vi "TXRX 5785 DDC DUC Measure Phase Stability.vi"() -> (0 "error out":errorcluster)   [LabVIEW 2019]
uses:
  <vilib>/userDefined/Silver/nirio_resource_slv.ctl
  <instrlib>/FlexRIO/API/Host/v1/NI FlexRIO/API/Reference Clock Source.ctl
  Common/Original 5785 Example/Host/Upconversion Mode.ctl
  <vilib>/Analysis/1siggen.llb/Ramp Pattern by Delta.vi
  <instrlib>/FlexRIO/API/Host/v1/NI FlexRIO/API/Configure Reference Clock.vi
  <instrlib>/FlexRIO/API/Host/v1/NI FlexRIO/API/Get Property Reference - Fpga Small.vi
  <instrlib>/FlexRIO/API/Host/v1/NI FlexRIO/API/Configure Analog Start Trigger.vi
  <instrlib>/FlexRIO/API/Host/v1/NI FlexRIO/API/Configure Digital Edge Start Trigger.vi
  <instrlib>/FlexRIO/API/Host/v1/NI FlexRIO/API/Configure Immediate Start Trigger.vi
  <instrlib>/FlexRIO/API/Host/v1/NI FlexRIO/API/Read Stream 1D WDT.vi
  <vilib>/measure/maspectr.llb/FFT Power Spectrum and PSD for N Chan.vi
  <vilib>/FPGAPlugInAG/Dynamic/niLvFpga_Close_Dynamic.vi
  <vilib>/Utility/file.llb/Write Delimited Spreadsheet (string).vi
  <vilib>/rvi/interface/nirviCloseFPGA/nirviCloseFPGA.xnode
  <instrlib>/FlexRIO/API/Host/v1/NI FlexRIO API v1.lvlib
  <resource>/objmgr/niflexrioapiStream.rc
  <vilib>/measure/NI_MAPro.lvlib
  Common/Original 5785 Example/Host/GettingStarted_5785_Host.lvlib
  <vilib>/Analysis/NI_AALPro.lvlib
  <vilib>/Analysis/NI_AALBase.lvlib
  <vilib>/measure/matone.llb/Extract Single Tone Information N Chan.vi
panel:
  out "Magnitude":cluster{"t0":dbl, "dt":dbl, "Y":dbl[]}(graph)={"t0"=0.0, "dt"=6.25e-10, "Y"=[0.00021584455710773213, 0.00043168911421546426, 0.00043168911421546426, 0.0004826431022662244, 0.00021584455710773213, 0.00021584455710773213, 0.0, 0.0003052503000261688, 0.00021584455710773213, 0.0003052503000261688, 0.0003052503000261688, 0.00021584455710773213, 0.0008899499076698426, 0.0004826431022662244, 0.00021584455710773213, 0.0004826431022662244, 0.00021584455710773213, 0.0004826431022662244, 0.00021584455710773213, 0.0006825604210107193, 0.00021584455710773213, 0.00021584455710773213, 0.0003052503000261688, 0.00021584455710773213, 0.00043168911421546426, 0.0004826431022662244, 0.0004826431022662244, 0.00043168911421546426, 0.0006825604210107193, 0.0004826431022662244, 0.00021584455710773213, 0.0006475336713231963, 0.00043168911421546426, 0.00021584455710773213, 0.0, 0.0003052503000261688, 0.0003052503000261688, 0.00021584455710773213, 0.0003052503000261688, 0.0003052503000261688, 0.0, 0.0, 0.00043168911421546426, 0.0004826431022662244, 0.00043168911421546426, 0.00043168911421546426, 0.0007782386181817434, 0.00021584455710773213, 0.00021584455710773213, 0.0003052503000261688, 0.00021584455710773213, 0.0, 0.00021584455710773213, 0.0003052503000261688, 0.00021584455710773213, 0.0004826431022662244, 0.00043168911421546426, 0.00043168911421546426, 0.0004826431022662244, 0.0003052503000261688, 0.0003052503000261688, 0.0004826431022662244, 0.0006825604210107193, 0.0004826431022662244, 0.00043168911421546426, 0.0003052503000261688, 0.0003052503000261688, 0.0003052503000261688, 0.00043168911421546426, 0.0004826431022662244, 0.0006825604210107193, 0.0003052503000261688, 0.0003052503000261688, 0.0, 0.00021584455710773213, 0.0003052503000261688, 0.0003052503000261688, 0.0004826431022662244, 0.0003052503000261688, 0.00021584455710773213, 0.00021584455710773213, 0.0011623585127480927, 0.0003052503000261688, 0.0006825604210107193, 0.00021584455710773213, 0.00021584455710773213, 0.00021584455710773213, 0.0006475336713231963, 0.0004826431022662244, 0.0004826431022662244, 0.0, 0.0003052503000261688, 0.00021584455710773213, 0.00021584455710773213, 0.00021584455710773213, 0.00021584455710773213, 0.0, 0.00021584455710773213, 0.00021584455710773213, 0.00043168911421546426, 0.0004826431022662244, 0.00021584455710773213, 0.0003052503000261688, 0.0, 0.00021584455710773213, 0.0003052503000261688, 0.0, 0.0003052503000261688, 0.0004826431022662244, 0.00021584455710773213, 0.0006105006000523376, 0.0003052503000261688, 0.00043168911421546426, 0.0, 0.00021584455710773213, 0.00043168911421546426, 0.0003052503000261688, 0.0, 0.00043168911421546426, 0.00021584455710773213, 0.0003052503000261688, 0.00021584455710773213, 0.00021584455710773213, 0.0004826431022662244, 0.0006105006000523376, 0.0003052503000261688, 0.0006105006000523376, 0.00021584455710773213, 0.0, 0.0004826431022662244, 0.00021584455710773213, 0.00021584455710773213, 0.0003052503000261688, 0.00021584455710773213, 0.00021584455710773213, 0.0004826431022662244, 0.00021584455710773213, 0.0004826431022662244, 0.00021584455710773213, 0.0004826431022662244, 0.0003052503000261688, 0.0, 0.0007782386181817434, 0.00021584455710773213, 0.00021584455710773213, 0.00043168911421546426, 0.00021584455710773213, 0.0, 0.00021584455710773213, 0.00021584455710773213, 0.00021584455710773213, 0.0003052503000261688, 0.00021584455710773213, 0.00043168911421546426, 0.0004826431022662244, 0.00021584455710773213, 0.0004826431022662244, 0.0003052503000261688, 0.0004826431022662244, 0.0003052503000261688, 0.0, 0.00021584455710773213, 0.00021584455710773213, 0.00043168911421546426, 0.0003052503000261688, 0.00021584455710773213, 0.0004826431022662244, 0.0003052503000261688, 0.00021584455710773213, 0.0, 0.0003052503000261688, 0.0004826431022662244, 0.0006825604210107193, 0.0, 0.00021584455710773213, 0.0, 0.0, 0.0, 0.0003052503000261688, 0.00021584455710773213, 0.00043168911421546426, 0.0004826431022662244, 0.0, 0.00021584455710773213, 0.0006105006000523376, 0.0004826431022662244, 0.00021584455710773213, 0.00021584455710773213, 0.0003052503000261688, 0.0003052503000261688, 0.0004826431022662244, 0.0, 0.00043168911421546426, 0.0004826431022662244, 0.00021584455710773213, 0.0003052503000261688, 0.0, 0.0, 0.00021584455710773213, 0.00021584455710773213, 0.00021584455710773213, 0.00021584455710773213, 0.0003052503000261688, 0.00021584455710773213, 0.00021584455710773213, 0.00021584455710773213, 0.0003052503000261688, 0.0003052503000261688, 0.00021584455710773213, 0.00021584455710773213, 0.00043168911421546426, 0.00021584455710773213, 0.0003052503000261688, 0.00021584455710773213, 0.0006475336713231963, 0.0, 0.0003052503000261688, 0.00021584455710773213, 0.0, 0.00021584455710773213, 0.00021584455710773213, 0.00021584455710773213, 0.00021584455710773213, 0.00043168911421546426, 0.0003052503000261688, 0.0006475336713231963, 0.0, 0.00043168911421546426, 0.0006475336713231963, 0.0003052503000261688, 0.0006825604210107193, 0.0003052503000261688, 0.0003052503000261688, 0.00021584455710773213, 0.0, 0.0003052503000261688, 0.0004826431022662244, 0.00021584455710773213, 0.0004826431022662244, 0.0006825604210107193, 0.00021584455710773213, 0.00043168911421546426, 0.00021584455710773213, 0.00021584455710773213, 0.0006475336713231963, 0.00021584455710773213, 0.0004826431022662244, 0.00021584455710773213, 0.0, 0.0008899499076698426, 0.00021584455710773213, 0.00043168911421546426, 0.0006105006000523376, 0.00021584455710773213, 0.0006105006000523376, 0.0003052503000261688, 0.00021584455710773213, 0.0006475336713231963, 0.0003052503000261688, 0.0003052503000261688, 0.0003052503000261688, 0.00021584455710773213, 0.0003052503000261688, 0.0003052503000261688, 0.0004826431022662244, 0.00021584455710773213, 0.00021584455710773213, 0.00043168911421546426, 0.00043168911421546426, 0.00021584455710773213, 0.0, 0.00021584455710773213, 0.00021584455710773213, 0.00043168911421546426, 0.0003052503000261688, 0.00021584455710773213, 0.00021584455710773213, 0.00043168911421546426, 0.0003052503000261688, 0.00043168911421546426, 0.00021584455710773213, 0.00021584455710773213, 0.0004826431022662244, 0.0004826431022662244, 0.00043168911421546426, 0.00021584455710773213, 0.00021584455710773213, 0.0003052503000261688, 0.0, 0.0, 0.00043168911421546426, 0.0003052503000261688, 0.00021584455710773213, 0.0004826431022662244, 0.00021584455710773213, 0.0, 0.00021584455710773213, 0.00021584455710773213, 0.00021584455710773213, 0.00043168911421546426, 0.0004826431022662244, 0.0003052503000261688, 0.00043168911421546426, 0.0003052503000261688, 0.00021584455710773213, 0.0, 0.00021584455710773213, 0.0003052503000261688, 0.0, 0.00021584455710773213, 0.0004826431022662244, 0.0009157509000785064, 0.00021584455710773213, 0.0007782386181817434, 0.00021584455710773213, 0.0, 0.00021584455710773213, 0.0003052503000261688, 0.00043168911421546426, 0.0004826431022662244, 0.0003052503000261688, 0.00021584455710773213, 0.0003052503000261688, 0.00021584455710773213, 0.00021584455710773213, 0.0, 0.0003052503000261688, 0.0003052503000261688, 0.00021584455710773213, 0.0003052503000261688, 0.00021584455710773213, 0.00043168911421546426, 0.00043168911421546426, 0.0003052503000261688, 0.0003052503000261688, 0.00021584455710773213, 0.00021584455710773213, 0.0003052503000261688, 0.00021584455710773213, 0.00021584455710773213, 0.0003052503000261688, 0.0003052503000261688, 0.0004826431022662244, 0.00021584455710773213, 0.0004826431022662244, 0.0004826431022662244, 0.00021584455710773213, 0.00043168911421546426, 0.0004826431022662244, 0.0004826431022662244, 0.0003052503000261688, 0.00043168911421546426, 0.00043168911421546426, 0.0006825604210107193, 0.00021584455710773213, 0.00021584455710773213, 0.0, 0.0004826431022662244, 0.00043168911421546426, 0.00021584455710773213, 0.0, 0.0003052503000261688, 0.00021584455710773213, 0.00043168911421546426, 0.0003052503000261688, 0.00021584455710773213, 0.0006825604210107193, 0.00021584455710773213, 0.00021584455710773213, 0.00021584455710773213, 0.00021584455710773213, 0.0003052503000261688, 0.0004826431022662244, 0.00021584455710773213, 0.0, 0.00021584455710773213, 0.0003052503000261688, 0.0004826431022662244, 0.0006475336713231963, 0.0003052503000261688, 0.00043168911421546426, 0.0, 0.0004826431022662244, 0.00021584455710773213, 0.0003052503000261688, 0.00021584455710773213, 0.0004826431022662244, 0.0003052503000261688, 0.00021584455710773213, 0.00021584455710773213, 0.0003052503000261688, 0.0003052503000261688, 0.0003052503000261688, 0.00043168911421546426, 0.0003052503000261688, 0.0, 0.00021584455710773213, 0.0003052503000261688, 0.00021584455710773213, 0.00021584455710773213, 0.0004826431022662244, 0.00043168911421546426, 0.00021584455710773213, 0.0003052503000261688, 0.0, 0.0003052503000261688, 0.0004826431022662244, 0.0003052503000261688, 0.00021584455710773213, 0.00021584455710773213, 0.00021584455710773213, 0.00021584455710773213, 0.00021584455710773213, 0.00021584455710773213, 0.0003052503000261688, 0.00021584455710773213, 0.0003052503000261688, 0.0003052503000261688, 0.0, 0.0, 0.0, 0.0003052503000261688, 0.00021584455710773213, 0.0004826431022662244, 0.0006475336713231963, 0.0006825604210107193, 0.00021584455710773213, 0.00021584455710773213, 0.00043168911421546426, 0.00021584455710773213, 0.00021584455710773213, 0.0003052503000261688, 0.0004826431022662244, 0.0004826431022662244, 0.00021584455710773213, 0.0, 0.0, 0.0003052503000261688, 0.0004826431022662244, 0.00021584455710773213, 0.0003052503000261688, 0.0004826431022662244, 0.00021584455710773213, 0.0003052503000261688, 0.00021584455710773213, 0.0003052503000261688, 0.0004826431022662244, 0.00021584455710773213, 0.0004826431022662244, 0.00021584455710773213, 0.0003052503000261688, 0.0003052503000261688, 0.0004826431022662244, 0.0, 0.00021584455710773213, 0.0, 0.00043168911421546426, 0.00043168911421546426, 0.0004826431022662244, 0.00043168911421546426, 0.00043168911421546426, 0.00021584455710773213, 0.00021584455710773213, 0.0004826431022662244, 0.00021584455710773213, 0.00021584455710773213, 0.00021584455710773213, 0.00021584455710773213, 0.00021584455710773213, 0.0004826431022662244, 0.0003052503000261688, 0.0004826431022662244, 0.0004826431022662244, 0.0006105006000523376, 0.0003052503000261688, 0.0, 0.0003052503000261688, 0.0003052503000261688, 0.0004826431022662244, 0.0004826431022662244, 0.00043168911421546426, 0.0004826431022662244, 0.0, 0.0, 0.0003052503000261688, 0.0003052503000261688, 0.0, 0.00021584455710773213, 0.00021584455710773213, 0.0003052503000261688, 0.00021584455710773213, 0.0003052503000261688, 0.00021584455710773213, 0.0003052503000261688, 0.00021584455710773213, 0.0003052503000261688, 0.00043168911421546426, 0.0004826431022662244, 0.00021584455710773213, 0.0003052503000261688, 0.00021584455710773213, 0.0003052503000261688, 0.0003052503000261688, 0.00021584455710773213, 0.00043168911421546426, 0.0003052503000261688, 0.0, 0.00021584455710773213, 0.0004826431022662244, 0.0003052503000261688, 0.0006105006000523376, 0.00021584455710773213, 0.0004826431022662244, 0.00021584455710773213, 0.00021584455710773213, 0.00021584455710773213, 0.0, 0.00021584455710773213, 0.0004826431022662244, 0.00021584455710773213, 0.0003052503000261688, 0.00021584455710773213, 0.0006825604210107193, 0.0003052503000261688, 0.0003052503000261688, 0.0003052503000261688, 0.0003052503000261688, 0.00021584455710773213, 0.0003052503000261688, 0.0, 0.00043168911421546426, 0.0003052503000261688, 0.0003052503000261688, 0.0003052503000261688, 0.00021584455710773213, 0.0003052503000261688, 0.0003052503000261688, 0.00043168911421546426, 0.0003052503000261688, 0.0003052503000261688, 0.0004826431022662244, 0.00021584455710773213, 0.0, 0.0003052503000261688, 0.0003052503000261688, 0.0004826431022662244, 0.00043168911421546426, 0.0003052503000261688, 0.00021584455710773213, 0.0, 0.0006105006000523376, 0.0004826431022662244, 0.00021584455710773213, 0.00021584455710773213, 0.0003052503000261688, 0.0004826431022662244, 0.0003052503000261688, 0.00043168911421546426, 0.0003052503000261688, 0.0004826431022662244, 0.0003052503000261688, 0.0006825604210107193, 0.0, 0.00021584455710773213, 0.0003052503000261688, 0.00021584455710773213, 0.0, 0.0, 0.00021584455710773213, 0.00021584455710773213, 0.0, 0.0004826431022662244, 0.0003052503000261688, 0.00021584455710773213, 0.0, 0.0, 0.00021584455710773213, 0.0003052503000261688, 0.0003052503000261688, 0.00021584455710773213, 0.00021584455710773213, 0.0004826431022662244, 0.00021584455710773213, 0.0003052503000261688, 0.00021584455710773213, 0.0004826431022662244, 0.00021584455710773213, 0.0004826431022662244, 0.0003052503000261688, 0.00021584455710773213, 0.0, 0.0003052503000261688, 0.0003052503000261688, 0.0003052503000261688, 0.0, 0.00043168911421546426, 0.0004826431022662244, 0.0, 0.0003052503000261688, 0.00021584455710773213, 0.0006105006000523376, 0.0004826431022662244, 0.00021584455710773213, 0.0003052503000261688, 0.0003052503000261688, 0.0003052503000261688, 0.0, 0.0003052503000261688, 0.0004826431022662244, 0.00021584455710773213, 0.00021584455710773213, 0.0004826431022662244, 0.00043168911421546426, 0.0, 0.0004826431022662244, 0.00021584455710773213, 0.0003052503000261688, 0.0, 0.00021584455710773213, 0.00021584455710773213, 0.0003052503000261688, 0.0003052503000261688, 0.00021584455710773213, 0.00043168911421546426, 0.00021584455710773213, 0.00021584455710773213, 0.0004826431022662244, 0.0003052503000261688, 0.0004826431022662244, 0.0004826431022662244, 0.00021584455710773213, 0.0004826431022662244, 0.00021584455710773213, 0.0, 0.0006475336713231963, 0.0, 0.00021584455710773213, 0.0, 0.0004826431022662244, 0.00043168911421546426, 0.0, 0.0, 0.0006105006000523376, 0.00021584455710773213, 0.00021584455710773213, 0.0003052503000261688, 0.0004826431022662244, 0.00021584455710773213, 0.0003052503000261688, 0.0, 0.0003052503000261688, 0.0004826431022662244, 0.0004826431022662244, 0.0004826431022662244, 0.0004826431022662244, 0.0004826431022662244, 0.00021584455710773213, 0.0, 0.00021584455710773213, 0.00021584455710773213, 0.00021584455710773213, 0.0004826431022662244, 0.00021584455710773213, 0.0003052503000261688, 0.0003052503000261688, 0.00043168911421546426, 0.00021584455710773213, 0.0003052503000261688, 0.0004826431022662244, 0.0003052503000261688, 0.0003052503000261688, 0.00043168911421546426, 0.00021584455710773213, 0.0003052503000261688, 0.0004826431022662244, 0.0003052503000261688, 0.0006825604210107193, 0.00043168911421546426, 0.00021584455710773213, 0.0003052503000261688, 0.0003052503000261688, 0.00021584455710773213, 0.0, 0.00021584455710773213, 0.0003052503000261688, 0.0, 0.0004826431022662244, 0.00021584455710773213, 0.00021584455710773213, 0.0004826431022662244, 0.00021584455710773213, 0.0003052503000261688, 0.00021584455710773213, 0.0003052503000261688, 0.00021584455710773213, 0.00021584455710773213, 0.0003052503000261688, 0.00021584455710773213, 0.00021584455710773213, 0.00043168911421546426, 0.0008899499076698426, 0.0004826431022662244, 0.00021584455710773213, 0.00021584455710773213, 0.0004826431022662244, 0.00043168911421546426, 0.0003052503000261688, 0.00043168911421546426, 0.00021584455710773213, 0.0, 0.0003052503000261688, 0.0006105006000523376, 0.00043168911421546426, 0.0003052503000261688, 0.00021584455710773213, 0.00021584455710773213, 0.00021584455710773213, 0.00021584455710773213, 0.0004826431022662244, 0.00021584455710773213, 0.00021584455710773213, 0.00021584455710773213, 0.0004826431022662244, 0.00021584455710773213, 0.00021584455710773213, 0.00021584455710773213, 0.0003052503000261688, 0.0003052503000261688, 0.00021584455710773213, 0.00021584455710773213, 0.00021584455710773213, 0.0004826431022662244, 0.00043168911421546426, 0.00021584455710773213, 0.0, 0.0, 0.0, 0.00021584455710773213, 0.0, 0.0003052503000261688, 0.00021584455710773213, 0.0004826431022662244, 0.0006825604210107193, 0.0006825604210107193, 0.0003052503000261688, 0.0003052503000261688, 0.0003052503000261688, 0.0006825604210107193, 0.0003052503000261688, 0.00021584455710773213, 0.0004826431022662244, 0.0004826431022662244, 0.0003052503000261688, 0.0004826431022662244, 0.00043168911421546426, 0.00021584455710773213, 0.00021584455710773213, 0.00021584455710773213, 0.00043168911421546426, 0.0006475336713231963, 0.0003052503000261688, 0.00021584455710773213, 0.0003052503000261688, 0.0, 0.00021584455710773213, 0.00043168911421546426, 0.0004826431022662244, 0.0003052503000261688, 0.0004826431022662244, 0.0006825604210107193, 0.0003052503000261688, 0.00021584455710773213, 0.00043168911421546426, 0.0003052503000261688, 0.0003052503000261688, 0.0003052503000261688, 0.0006475336713231963, 0.00043168911421546426, 0.00021584455710773213, 0.0003052503000261688, 0.0003052503000261688, 0.0004826431022662244, 0.0004826431022662244, 0.0003052503000261688, 0.0003052503000261688, 0.0006105006000523376, 0.0003052503000261688, 0.00043168911421546426, 0.00021584455710773213, 0.0003052503000261688, 0.0003052503000261688, 0.0, 0.00021584455710773213, 0.0004826431022662244, 0.00021584455710773213, 0.00021584455710773213, 0.0003052503000261688, 0.00021584455710773213, 0.0003052503000261688, 0.0003052503000261688, 0.0004826431022662244, 0.0, 0.0004826431022662244, 0.0003052503000261688, 0.0003052503000261688, 0.0, 0.00021584455710773213, 0.0004826431022662244, 0.0006105006000523376, 0.0006105006000523376, 0.0003052503000261688, 0.00021584455710773213, 0.0004826431022662244, 0.0003052503000261688, 0.0004826431022662244, 0.00021584455710773213, 0.0003052503000261688, 0.0003052503000261688, 0.0, 0.0004826431022662244, 0.00021584455710773213, 0.0003052503000261688, 0.0006105006000523376, 0.0003052503000261688, 0.0006825604210107193, 0.00021584455710773213, 0.00021584455710773213, 0.0, 0.00043168911421546426, 0.0006105006000523376, 0.0004826431022662244, 0.0003052503000261688, 0.0004826431022662244, 0.0003052503000261688, 0.0004826431022662244, 0.00043168911421546426, 0.00043168911421546426, 0.00021584455710773213, 0.0004826431022662244, 0.00021584455710773213, 0.00021584455710773213, 0.0003052503000261688, 0.00021584455710773213, 0.00021584455710773213, 0.0006475336713231963, 0.0004826431022662244, 0.00043168911421546426, 0.0, 0.0, 0.0006825604210107193, 0.00021584455710773213, 0.00043168911421546426, 0.0, 0.00043168911421546426, 0.00021584455710773213, 0.0, 0.0006105006000523376, 0.0004826431022662244, 0.00043168911421546426, 0.00043168911421546426, 0.00043168911421546426, 0.0004826431022662244, 0.00043168911421546426, 0.0004826431022662244, 0.00021584455710773213, 0.0, 0.00021584455710773213, 0.0, 0.00043168911421546426, 0.0, 0.00021584455710773213, 0.0003052503000261688, 0.00021584455710773213, 0.00021584455710773213, 0.0003052503000261688, 0.0003052503000261688, 0.00021584455710773213, 0.00021584455710773213, 0.0004826431022662244, 0.0, 0.0003052503000261688, 0.0003052503000261688, 0.0003052503000261688, 0.0003052503000261688, 0.00043168911421546426, 0.0004826431022662244, 0.0004826431022662244, 0.00021584455710773213, 0.0003052503000261688, 0.0004826431022662244, 0.00021584455710773213, 0.0, 0.00021584455710773213, 0.00021584455710773213, 0.0003052503000261688, 0.0003052503000261688, 0.00021584455710773213, 0.00021584455710773213, 0.0003052503000261688, 0.00043168911421546426, 0.00043168911421546426, 0.0003052503000261688, 0.00021584455710773213, 0.0006825604210107193, 0.0006105006000523376, 0.0007782386181817434, 0.0003052503000261688, 0.0003052503000261688, 0.00021584455710773213, 0.0003052503000261688, 0.00043168911421546426, 0.00021584455710773213, 0.00021584455710773213, 0.00043168911421546426, 0.00021584455710773213, 0.0, 0.0006825604210107193, 0.00021584455710773213, 0.00043168911421546426, 0.0004826431022662244, 0.0003052503000261688, 0.0009652862045324488, 0.00021584455710773213, 0.0004826431022662244, 0.00021584455710773213, 0.0003052503000261688, 0.0003052503000261688, 0.00021584455710773213, 0.0, 0.00021584455710773213, 0.0, 0.00021584455710773213, 0.0004826431022662244, 0.0004826431022662244, 0.0, 0.0003052503000261688, 0.00021584455710773213, 0.00043168911421546426, 0.00021584455710773213, 0.0003052503000261688, 0.0004826431022662244, 0.0006105006000523376, 0.0, 0.0003052503000261688, 0.00021584455710773213, 0.00021584455710773213, 0.00021584455710773213, 0.0003052503000261688, 0.0003052503000261688, 0.00021584455710773213, 0.0003052503000261688, 0.00043168911421546426, 0.0004826431022662244, 0.00021584455710773213, 0.0003052503000261688, 0.0004826431022662244, 0.0003052503000261688, 0.0003052503000261688, 0.0003052503000261688, 0.0003052503000261688, 0.0004826431022662244, 0.00021584455710773213, 0.0003052503000261688, 0.0003052503000261688, 0.00021584455710773213, 0.00021584455710773213, 0.00043168911421546426, 0.00021584455710773213, 0.0, 0.0003052503000261688, 0.0, 0.0, 0.00043168911421546426, 0.0004826431022662244, 0.0003052503000261688, 0.00021584455710773213, 0.0003052503000261688, 0.00021584455710773213, 0.0003052503000261688, 0.0004826431022662244, 0.00021584455710773213, 0.00021584455710773213, 0.00021584455710773213, 0.00021584455710773213, 0.00021584455710773213, 0.0004826431022662244, 0.00043168911421546426, 0.0006825604210107193, 0.0003052503000261688, 0.00021584455710773213, 0.00021584455710773213, 0.00021584455710773213, 0.00021584455710773213, 0.0003052503000261688, 0.0, 0.0, 0.0003052503000261688, 0.0006475336713231963, 0.0003052503000261688, 0.0003052503000261688, 0.0003052503000261688, 0.0, 0.0, 0.00021584455710773213, 0.0003052503000261688, 0.0003052503000261688, 0.0006825604210107193, 0.0003052503000261688, 0.0004826431022662244, 0.0006475336713231963, 0.0006105006000523376, 0.00021584455710773213, 0.0, 0.0004826431022662244, 0.0003052503000261688, 0.00021584455710773213, 0.0003052503000261688, 0.0003052503000261688, 0.00021584455710773213, 0.00043168911421546426, 0.00021584455710773213, 0.0006475336713231963, 0.0, 0.00021584455710773213]}
  in  "Remove Frequency Offset":bool
  out "Amplitude Stability":dbl=-75.28004784677937 format="%.6p"
  out "Phase Stability":dbl=6.266755784750002 format="%.6p"
  out "Phase":cluster{"t0":dbl, "dt":dbl, "Y":dbl[]}(graph)={"t0"=0.0, "dt"=6.25e-10, "Y"=[-1.5707963267948966, 3.141592653589793, 1.5707963267948966, -1.1071487177940904, 0.0, 0.0, 0.0, 2.356194490192345, -1.5707963267948966, -2.356194490192345, -0.7853981633974483, 3.141592653589793, -1.8157749899217608, -2.0344439357957027, 1.5707963267948966, 2.0344439357957027, -1.5707963267948966, -2.677945044588987, 1.5707963267948966, -1.2490457723982544, 3.141592653589793, -1.5707963267948966, 0.7853981633974483, 3.141592653589793, -1.5707963267948966, -2.0344439357957027, 1.1071487177940904, -1.5707963267948966, 2.819842099193151, -2.0344439357957027, 3.141592653589793, 3.141592653589793, 3.141592653589793, 3.141592653589793, 0.0, -2.356194490192345, -0.7853981633974483, 3.141592653589793, -2.356194490192345, 2.356194490192345, 0.0, 0.0, -1.5707963267948966, -1.1071487177940904, 3.141592653589793, 0.0, -2.158798930342464, 3.141592653589793, -1.5707963267948966, -2.356194490192345, 1.5707963267948966, 0.0, 0.0, -0.7853981633974483, -1.5707963267948966, -2.0344439357957027, 3.141592653589793, 3.141592653589793, -2.0344439357957027, -0.7853981633974483, -2.356194490192345, -0.4636476090008061, -1.892546881191539, 2.0344439357957027, 0.0, -2.356194490192345, -2.356194490192345, -2.356194490192345, 3.141592653589793, -0.4636476090008061, -1.892546881191539, 2.356194490192345, -0.7853981633974483, 0.0, 3.141592653589793, 2.356194490192345, -2.356194490192345, -2.0344439357957027, 2.356194490192345, 3.141592653589793, 0.0, -2.761086276477428, 0.7853981633974483, -1.2490457723982544, 3.141592653589793, -1.5707963267948966, 3.141592653589793, 3.141592653589793, -2.0344439357957027, -2.0344439357957027, 0.0, -2.356194490192345, 3.141592653589793, 3.141592653589793, -1.5707963267948966, -1.5707963267948966, 0.0, 3.141592653589793, 1.5707963267948966, -1.5707963267948966, -2.677945044588987, -1.5707963267948966, -2.356194490192345, 0.0, 3.141592653589793, -2.356194490192345, 0.0, -0.7853981633974483, 2.677945044588987, -1.5707963267948966, -2.356194490192345, -2.356194490192345, 3.141592653589793, 0.0, 1.5707963267948966, -1.5707963267948966, 2.356194490192345, 0.0, -1.5707963267948966, -1.5707963267948966, -2.356194490192345, -1.5707963267948966, 3.141592653589793, -2.677945044588987, -2.356194490192345, -0.7853981633974483, -2.356194490192345, 1.5707963267948966, 0.0, -2.677945044588987, 1.5707963267948966, -1.5707963267948966, -2.356194490192345, -1.5707963267948966, 3.141592653589793, -2.677945044588987, -1.5707963267948966, -2.677945044588987, 1.5707963267948966, -2.677945044588987, -2.356194490192345, 0.0, -2.158798930342464, 3.141592653589793, 0.0, 3.141592653589793, 1.5707963267948966, 0.0, 0.0, 3.141592653589793, 3.141592653589793, -2.356194490192345, -1.5707963267948966, 3.141592653589793, 1.1071487177940904, -1.5707963267948966, -2.677945044588987, -2.356194490192345, -2.0344439357957027, 2.356194490192345, 0.0, 0.0, -1.5707963267948966, -1.5707963267948966, -2.356194490192345, 0.0, -2.0344439357957027, 2.356194490192345, 3.141592653589793, 0.0, -2.356194490192345, 2.677945044588987, -2.819842099193151, 0.0, 3.141592653589793, 0.0, 0.0, 0.0, 2.356194490192345, -1.5707963267948966, 3.141592653589793, -2.677945044588987, 0.0, 3.141592653589793, -0.7853981633974483, -2.0344439357957027, 1.5707963267948966, 3.141592653589793, -2.356194490192345, -2.356194490192345, -2.0344439357957027, 0.0, 3.141592653589793, -2.0344439357957027, -1.5707963267948966, 2.356194490192345, 0.0, 0.0, 1.5707963267948966, 1.5707963267948966, 0.0, -1.5707963267948966, -0.7853981633974483, 1.5707963267948966, -1.5707963267948966, -1.5707963267948966, -2.356194490192345, -0.7853981633974483, 0.0, -1.5707963267948966, -1.5707963267948966, 3.141592653589793, -2.356194490192345, -1.5707963267948966, -1.5707963267948966, 0.0, -2.356194490192345, -1.5707963267948966, 0.0, 3.141592653589793, 0.0, -1.5707963267948966, 0.0, 3.141592653589793, -0.7853981633974483, 3.141592653589793, 0.0, -1.5707963267948966, 3.141592653589793, -0.7853981633974483, -1.892546881191539, 2.356194490192345, -2.356194490192345, -1.5707963267948966, 0.0, -2.356194490192345, -2.677945044588987, -1.5707963267948966, -2.0344439357957027, 2.819842099193151, -1.5707963267948966, 3.141592653589793, -1.5707963267948966, -1.5707963267948966, 3.141592653589793, 0.0, -2.0344439357957027, 3.141592653589793, 0.0, 2.896613990462929, 1.5707963267948966, -1.5707963267948966, -2.356194490192345, -1.5707963267948966, -2.356194490192345, 2.356194490192345, 0.0, 3.141592653589793, 2.356194490192345, -2.356194490192345, -2.356194490192345, 1.5707963267948966, -2.356194490192345, 2.356194490192345, -1.1071487177940904, -1.5707963267948966, 1.5707963267948966, -1.5707963267948966, 3.141592653589793, -1.5707963267948966, 0.0, 3.141592653589793, -1.5707963267948966, 3.141592653589793, -2.356194490192345, 1.5707963267948966, 0.0, 3.141592653589793, 2.356194490192345, -1.5707963267948966, -1.5707963267948966, -1.5707963267948966, -2.0344439357957027, 2.677945044588987, 3.141592653589793, 3.141592653589793, -1.5707963267948966, 0.7853981633974483, 0.0, 0.0, 3.141592653589793, -2.356194490192345, 0.0, -2.677945044588987, -1.5707963267948966, 0.0, -1.5707963267948966, -1.5707963267948966, 1.5707963267948966, -1.5707963267948966, 2.677945044588987, -0.7853981633974483, -1.5707963267948966, 2.356194490192345, 3.141592653589793, 0.0, -1.5707963267948966, -0.7853981633974483, 0.0, 0.0, -2.0344439357957027, 2.356194490192345, -1.5707963267948966, -2.5535900500422257, -1.5707963267948966, 0.0, -1.5707963267948966, -2.356194490192345, 3.141592653589793, -2.0344439357957027, 2.356194490192345, 3.141592653589793, -2.356194490192345, -1.5707963267948966, 3.141592653589793, 0.0, -2.356194490192345, -2.356194490192345, 3.141592653589793, -2.356194490192345, 0.0, -1.5707963267948966, 3.141592653589793, 0.7853981633974483, -2.356194490192345, 3.141592653589793, 3.141592653589793, -2.356194490192345, -1.5707963267948966, 3.141592653589793, -2.356194490192345, -0.7853981633974483, -2.0344439357957027, 3.141592653589793, -1.1071487177940904, -2.0344439357957027, 3.141592653589793, 3.141592653589793, -1.1071487177940904, -2.677945044588987, 0.7853981633974483, -1.5707963267948966, 3.141592653589793, -2.819842099193151, 1.5707963267948966, 0.0, 0.0, -1.1071487177940904, -1.5707963267948966, 3.141592653589793, 0.0, -2.356194490192345, 0.0, -1.5707963267948966, -2.356194490192345, 0.0, -1.892546881191539, -1.5707963267948966, 3.141592653589793, -1.5707963267948966, 0.0, -2.356194490192345, -1.1071487177940904, -1.5707963267948966, 0.0, 1.5707963267948966, -0.7853981633974483, -2.677945044588987, 1.5707963267948966, -2.356194490192345, 3.141592653589793, 0.0, -2.0344439357957027, 3.141592653589793, -2.356194490192345, -1.5707963267948966, -2.0344439357957027, 2.356194490192345, 0.0, 1.5707963267948966, -2.356194490192345, -2.356194490192345, -2.356194490192345, 3.141592653589793, 2.356194490192345, 0.0, -1.5707963267948966, -2.356194490192345, 1.5707963267948966, -1.5707963267948966, -2.677945044588987, -1.5707963267948966, -1.5707963267948966, 2.356194490192345, 0.0, 2.356194490192345, -2.0344439357957027, 2.356194490192345, 3.141592653589793, 1.5707963267948966, 3.141592653589793, -1.5707963267948966, 3.141592653589793, 0.0, -2.356194490192345, -1.5707963267948966, -0.7853981633974483, -2.356194490192345, 0.0, 0.0, 0.0, -2.356194490192345, 3.141592653589793, 2.677945044588987, -1.5707963267948966, -1.2490457723982544, -1.5707963267948966, 3.141592653589793, 3.141592653589793, -1.5707963267948966, 0.0, -2.356194490192345, -2.677945044588987, 2.677945044588987, 1.5707963267948966, 0.0, 0.0, -2.356194490192345, -2.0344439357957027, 3.141592653589793, -2.356194490192345, -2.0344439357957027, 3.141592653589793, -2.356194490192345, 3.141592653589793, -0.7853981633974483, -1.1071487177940904, 3.141592653589793, -2.677945044588987, 3.141592653589793, 0.7853981633974483, -2.356194490192345, -2.677945044588987, 0.0, -1.5707963267948966, 0.0, -1.5707963267948966, 3.141592653589793, 2.677945044588987, 3.141592653589793, 3.141592653589793, 3.141592653589793, 0.0, -1.1071487177940904, -1.5707963267948966, 3.141592653589793, 3.141592653589793, 3.141592653589793, -1.5707963267948966, -2.0344439357957027, -0.7853981633974483, 2.0344439357957027, -2.677945044588987, -2.356194490192345, 0.7853981633974483, 0.0, -2.356194490192345, -2.356194490192345, -2.677945044588987, -2.677945044588987, -1.5707963267948966, -2.677945044588987, 0.0, 0.0, -0.7853981633974483, -2.356194490192345, 0.0, -1.5707963267948966, 3.141592653589793, -2.356194490192345, 3.141592653589793, 2.356194490192345, 3.141592653589793, -0.7853981633974483, -1.5707963267948966, -2.356194490192345, -1.5707963267948966, -2.0344439357957027, 3.141592653589793, -2.356194490192345, 3.141592653589793, -2.356194490192345, -2.356194490192345, 3.141592653589793, 3.141592653589793, -2.356194490192345, 0.0, -1.5707963267948966, -2.677945044588987, -2.356194490192345, -2.356194490192345, 0.0, 1.1071487177940904, -1.5707963267948966, 0.0, -1.5707963267948966, 0.0, 0.0, -2.0344439357957027, 3.141592653589793, -0.7853981633974483, -1.5707963267948966, -1.892546881191539, 2.356194490192345, -0.7853981633974483, -2.356194490192345, -2.356194490192345, -1.5707963267948966, 2.356194490192345, 0.0, -1.5707963267948966, -0.7853981633974483, -0.7853981633974483, -2.356194490192345, 3.141592653589793, -2.356194490192345, 0.7853981633974483, 3.141592653589793, 0.7853981633974483, -2.356194490192345, -2.677945044588987, 3.141592653589793, 0.0, 2.356194490192345, -2.356194490192345, -2.677945044588987, 3.141592653589793, -2.356194490192345, 3.141592653589793, 0.0, -2.356194490192345, 2.677945044588987, 3.141592653589793, 3.141592653589793, 0.7853981633974483, -1.1071487177940904, -2.356194490192345, -1.5707963267948966, 2.356194490192345, -2.677945044588987, -0.7853981633974483, -2.819842099193151, 0.0, -1.5707963267948966, -0.7853981633974483, -1.5707963267948966, 0.0, 0.0, -1.5707963267948966, -1.5707963267948966, 0.0, -2.0344439357957027, -2.356194490192345, 0.0, 0.0, 0.0, 3.141592653589793, -2.356194490192345, -2.356194490192345, -1.5707963267948966, 3.141592653589793, -2.677945044588987, 3.141592653589793, 2.356194490192345, 0.0, -1.1071487177940904, -1.5707963267948966, 2.677945044588987, -2.356194490192345, -1.5707963267948966, 0.0, -2.356194490192345, -2.356194490192345, -2.356194490192345, 0.0, -1.5707963267948966, -2.677945044588987, 0.0, -2.356194490192345, 3.141592653589793, -2.356194490192345, -2.0344439357957027, 3.141592653589793, -0.7853981633974483, 2.356194490192345, -0.7853981633974483, 0.0, -2.356194490192345, -1.1071487177940904, -1.5707963267948966, 3.141592653589793, -2.0344439357957027, 3.141592653589793, 0.0, -2.0344439357957027, 3.141592653589793, -0.7853981633974483, 0.0, 1.5707963267948966, 3.141592653589793, -2.356194490192345, -2.356194490192345, 3.141592653589793, -1.5707963267948966, 0.0, 1.5707963267948966, -2.677945044588987, 2.356194490192345, -0.4636476090008061, -2.677945044588987, 1.5707963267948966, -2.0344439357957027, -1.5707963267948966, 0.0, -1.5707963267948966, 0.0, -1.5707963267948966, 0.0, -2.677945044588987, -1.5707963267948966, 0.0, 0.0, -2.356194490192345, 3.141592653589793, 3.141592653589793, -2.356194490192345, -2.677945044588987, -1.5707963267948966, 2.356194490192345, 0.0, -2.356194490192345, 2.677945044588987, -1.1071487177940904, -2.677945044588987, 2.677945044588987, -2.0344439357957027, 3.141592653589793, 0.0, 1.5707963267948966, -1.5707963267948966, 0.0, -2.677945044588987, 1.5707963267948966, -2.356194490192345, -0.7853981633974483, 3.141592653589793, 0.0, -0.7853981633974483, -2.677945044588987, -0.7853981633974483, -2.356194490192345, 3.141592653589793, -1.5707963267948966, -2.356194490192345, -2.0344439357957027, 2.356194490192345, -1.2490457723982544, -1.5707963267948966, 3.141592653589793, -2.356194490192345, -0.7853981633974483, 3.141592653589793, 0.0, -1.5707963267948966, -2.356194490192345, 0.0, -2.0344439357957027, 1.5707963267948966, 0.0, -2.0344439357957027, -1.5707963267948966, -2.356194490192345, 3.141592653589793, 0.7853981633974483, 0.0, -1.5707963267948966, -2.356194490192345, -1.5707963267948966, -1.5707963267948966, 3.141592653589793, 2.896613990462929, 0.4636476090008061, -1.5707963267948966, 3.141592653589793, -1.1071487177940904, 3.141592653589793, 2.356194490192345, -1.5707963267948966, -1.5707963267948966, 0.0, 0.7853981633974483, -0.7853981633974483, 3.141592653589793, 0.7853981633974483, 3.141592653589793, 1.5707963267948966, -1.5707963267948966, -1.5707963267948966, -2.0344439357957027, -1.5707963267948966, 0.0, -1.5707963267948966, -2.0344439357957027, 3.141592653589793, 0.0, 3.141592653589793, -2.356194490192345, -2.356194490192345, 3.141592653589793, 0.0, -1.5707963267948966, -2.0344439357957027, -1.5707963267948966, 3.141592653589793, 0.0, 0.0, 0.0, 1.5707963267948966, 0.0, -0.7853981633974483, 3.141592653589793, -2.677945044588987, -2.819842099193151, 2.819842099193151, -0.7853981633974483, -2.356194490192345, -2.356194490192345, -1.892546881191539, -2.356194490192345, 0.0, 2.677945044588987, -2.677945044588987, -2.356194490192345, -2.677945044588987, 3.141592653589793, 3.141592653589793, 1.5707963267948966, 3.141592653589793, 3.141592653589793, 3.141592653589793, -0.7853981633974483, 3.141592653589793, 0.7853981633974483, 0.0, -1.5707963267948966, 3.141592653589793, -2.677945044588987, 2.356194490192345, -0.4636476090008061, -2.819842099193151, -2.356194490192345, -1.5707963267948966, 3.141592653589793, 0.7853981633974483, -2.356194490192345, 2.356194490192345, -1.5707963267948966, -1.5707963267948966, 3.141592653589793, -2.356194490192345, -2.356194490192345, 0.4636476090008061, -2.0344439357957027, 2.356194490192345, -0.7853981633974483, -2.356194490192345, 0.7853981633974483, 1.5707963267948966, 0.0, -2.356194490192345, 0.7853981633974483, 0.0, -1.5707963267948966, -2.0344439357957027, 0.0, -1.5707963267948966, -2.356194490192345, -1.5707963267948966, -2.356194490192345, 2.356194490192345, -1.1071487177940904, 0.0, 2.677945044588987, -2.356194490192345, 2.356194490192345, 0.0, 3.141592653589793, 2.677945044588987, -0.7853981633974483, -2.356194490192345, 0.7853981633974483, -1.5707963267948966, -2.0344439357957027, -2.356194490192345, -2.0344439357957027, 1.5707963267948966, -2.356194490192345, -2.356194490192345, 0.0, -1.1071487177940904, 3.141592653589793, 0.7853981633974483, -2.356194490192345, 2.356194490192345, -1.2490457723982544, -1.5707963267948966, 3.141592653589793, 0.0, 3.141592653589793, -0.7853981633974483, -2.0344439357957027, 2.356194490192345, -0.4636476090008061, -2.356194490192345, -2.0344439357957027, -1.5707963267948966, 3.141592653589793, -1.5707963267948966, -2.0344439357957027, -1.5707963267948966, 3.141592653589793, -2.356194490192345, 1.5707963267948966, 3.141592653589793, 3.141592653589793, -0.4636476090008061, -1.5707963267948966, 0.0, 0.0, -2.819842099193151, 1.5707963267948966, -1.5707963267948966, 0.0, 3.141592653589793, -1.5707963267948966, 0.0, -0.7853981633974483, -2.677945044588987, 1.5707963267948966, -1.5707963267948966, 3.141592653589793, -2.0344439357957027, -1.5707963267948966, 2.0344439357957027, 3.141592653589793, 0.0, -1.5707963267948966, 0.0, 3.141592653589793, 0.0, 1.5707963267948966, -0.7853981633974483, 3.141592653589793, -1.5707963267948966, -2.356194490192345, -2.356194490192345, 0.0, 0.0, -1.1071487177940904, 0.0, -0.7853981633974483, -2.356194490192345, -2.356194490192345, -2.356194490192345, -1.5707963267948966, -1.1071487177940904, 0.4636476090008061, -1.5707963267948966, -2.356194490192345, -0.4636476090008061, -1.5707963267948966, 0.0, 3.141592653589793, 0.0, 2.356194490192345, -2.356194490192345, 3.141592653589793, 3.141592653589793, -2.356194490192345, -1.5707963267948966, 3.141592653589793, -0.7853981633974483, 3.141592653589793, 2.819842099193151, -0.7853981633974483, -2.5535900500422257, 0.7853981633974483, -0.7853981633974483, 3.141592653589793, -2.356194490192345, 3.141592653589793, 3.141592653589793, 3.141592653589793, -1.5707963267948966, -1.5707963267948966, 0.0, 2.819842099193151, 0.0, -1.5707963267948966, 2.0344439357957027, -0.7853981633974483, -2.677945044588987, 1.5707963267948966, -1.1071487177940904, 3.141592653589793, -2.356194490192345, -2.356194490192345, 3.141592653589793, 0.0, 1.5707963267948966, 0.0, 0.0, 2.677945044588987, -0.4636476090008061, 0.0, -2.356194490192345, -1.5707963267948966, -1.5707963267948966, 1.5707963267948966, -2.356194490192345, -2.677945044588987, -2.356194490192345, 0.0, -2.356194490192345, -1.5707963267948966, 0.0, 3.141592653589793, -2.356194490192345, 2.356194490192345, 1.5707963267948966, -2.356194490192345, -1.5707963267948966, 2.677945044588987, -1.5707963267948966, -0.7853981633974483, -2.0344439357957027, -2.356194490192345, -2.356194490192345, 0.7853981633974483, -2.356194490192345, -1.1071487177940904, 3.141592653589793, -2.356194490192345, -0.7853981633974483, 3.141592653589793, 3.141592653589793, 3.141592653589793, 3.141592653589793, 0.0, -2.356194490192345, 0.0, 0.0, -1.5707963267948966, -2.0344439357957027, -2.356194490192345, 3.141592653589793, 2.356194490192345, 3.141592653589793, -2.356194490192345, -2.0344439357957027, -1.5707963267948966, 3.141592653589793, -1.5707963267948966, -1.5707963267948966, -1.5707963267948966, -2.677945044588987, 1.5707963267948966, -1.892546881191539, -2.356194490192345, 0.0, -1.5707963267948966, 1.5707963267948966, 3.141592653589793, -2.356194490192345, 0.0, 0.0, 0.7853981633974483, 3.141592653589793, -2.356194490192345, -2.356194490192345, -2.356194490192345, 0.0, 0.0, -1.5707963267948966, -2.356194490192345, 2.356194490192345, -2.819842099193151, 2.356194490192345, -0.4636476090008061, 3.141592653589793, 2.356194490192345, 3.141592653589793, 0.0, -2.677945044588987, -2.356194490192345, -1.5707963267948966, -0.7853981633974483, -2.356194490192345, 1.5707963267948966, -1.5707963267948966, 0.0, 3.141592653589793, 0.0, 0.0]}
  out "error out 4":errorcluster
  in  "Results Base Path":path=path "C:/Repos/bsherman-sandbox/CogRF/5785 Measurements/TX RX Phase Stability With DUC DDC/Results"
  out "error out 3":errorcluster
  out "Results":T1(array[cluster])=[{"frequency (Hz)"=10000000.0, "mean skew"=-75.20318719354484, "skew std dev"=0.5901215042031069, "skew pk-pk"=1.8717754513188964, "skews"=[-75.07430702018954, -75.44809048216575, -75.80198718423274, -75.16506159969862, -75.74776258499699, -75.40117480946905, -75.74938200683876, -73.93021173291385, -74.5381472725637, -75.17574724237929]}, {"frequency (Hz)"=50000000.0, "mean skew"=-74.92115147529958, "skew std dev"=0.23757929946673909, "skew pk-pk"=0.7012097707384868, "skews"=[-74.72629943177984, -74.84853377834897, -75.17338839352433, -75.07414552929393, -74.53453236811035, -75.18988856872822, -74.69907620424898, -74.83822334232389, -75.23574213884883, -74.89168499778843]}, {"frequency (Hz)"=100000000.0, "mean skew"=-75.16539855804271, "skew std dev"=0.42164963831432206, "skew pk-pk"=1.4677776258774458, "skews"=[-75.23215436661192, -75.0027730067996, -75.44434007691336, -74.88230297114421, -74.8293021697705, -75.34418758162698, -74.32857019090186, -75.22285720496009, -75.7963478167793, -75.57115019491921]}, {"frequency (Hz)"=150000000.0, "mean skew"=-75.40939936616591, "skew std dev"=0.37252489801146915, "skew pk-pk"=1.0692368549535587, "skews"=[-75.06019035982966, -75.29802302921661, -75.49980027058739, -75.43797935848387, -75.34128586615623, -75.9847593485702, -76.0099263030783, -74.9910484870499, -75.53029119056228, -74.94068944812474]}, {"frequency (Hz)"=200000000.0, "mean skew"=-75.66125221649293, "skew std dev"=0.3523368600704349, "skew pk-pk"=1.199835324068161, "skews"=[-75.59953041036991, -75.79016710046115, -75.51269894874414, -75.53983030043885, -75.8493578489041, -75.89551553098826, -76.15451828116109, -74.95468295709293, -75.9951542202909, -75.32106656647782]}, {"frequency (Hz)"=250000000.0, "mean skew"=-75.12488606365496, "skew std dev"=0.6002677903631366, "skew pk-pk"=2.050870186544671, "skews"=[-75.53867067607365, -74.90080191219263, -75.52468555826523, -75.65833632378144, -75.0756648192859, -75.72668554805085, -75.29404529917352, -74.98088302824068, -73.67581536150618, -74.87327210997957]}, {"frequency (Hz)"=300000000.0, "mean skew"=-74.87939621124528, "skew std dev"=0.608078870398904, "skew pk-pk"=2.243386913788285, "skews"=[-74.46605782731459, -75.32102634414092, -74.68921864796258, -75.10360135764758, -75.93320603873018, -75.40834153046363, -74.7516029898691, -74.72261164554641, -74.70847660583593, -73.68981912494189]}, {"frequency (Hz)"=350000000.0, "mean skew"=-74.88765889976952, "skew std dev"=0.5494930629507502, "skew pk-pk"=1.6166910414614364, "skews"=[-75.51669371073311, -74.21497824425641, -74.6113946129877, -75.83166928571785, -75.0204110411821, -74.37576043400422, -74.3177898243675, -75.16119823356729, -74.58073248230232, -75.24596112857674]}, {"frequency (Hz)"=400000000.0, "mean skew"=-75.10371333811172, "skew std dev"=0.5716237525117893, "skew pk-pk"=1.73565569368958, "skews"=[-74.69225737014143, -74.00818954039673, -75.59052021166649, -74.71036544653393, -75.6039372981583, -75.47862608497864, -74.90081671408467, -75.56219491528184, -75.74384523408631, -74.74638056578898]}, {"frequency (Hz)"=450000000.0, "mean skew"=-75.02541252028026, "skew std dev"=0.5474902082088354, "skew pk-pk"=1.7813202116072233, "skews"=[-74.2590992085695, -75.10408013162802, -74.03309193655438, -74.81348464665602, -74.90022747649351, -75.12505167678941, -75.43890566155079, -75.38336180974133, -75.81441214816161, -75.38241050665783]}, {"frequency (Hz)"=500000000.0, "mean skew"=-74.87667556017743, "skew std dev"=0.4719833652834626, "skew pk-pk"=1.319241320466105, "skews"=[-74.36709345930412, -75.26338004294415, -75.19530959536014, -74.498970335564, -75.43126249391054, -74.98971593701795, -75.15862887718677, -74.11202117344443, -74.4468363539694, -75.30353733307284]}, {"frequency (Hz)"=550000000.0, "mean skew"=-74.81762844923378, "skew std dev"=0.8882928898266298, "skew pk-pk"=2.8412559558441473, "skews"=[-74.84342478713931, -75.27348478689453, -75.7122938104698, -73.86943787933875, -75.8000932256467, -75.60964464486774, -74.54580255168042, -72.95883726980256, -74.96805214697734, -74.59521338952062]}, {"frequency (Hz)"=600000000.0, "mean skew"=-75.25881357115892, "skew std dev"=0.5037965199781086, "skew pk-pk"=1.7900335654313864, "skews"=[-75.2800192629812, -75.23991508354649, -75.32261471507837, -75.14642857620619, -74.00826764144773, -75.5772132716813, -75.79830120687912, -75.73302537754631, -75.03501862614887, -75.44733195007366]}, {"frequency (Hz)"=650000000.0, "mean skew"=-75.19515737079529, "skew std dev"=0.4586416954317144, "skew pk-pk"=1.5097515924690015, "skews"=[-75.1711650103267, -75.00582531913341, -74.9998713726656, -75.67405615662898, -75.07038266577976, -75.57381029926576, -75.74037957675006, -74.9279181222225, -74.23062798428106, -75.55753720089903]}, {"frequency (Hz)"=700000000.0, "mean skew"=-74.9593574847269, "skew std dev"=0.5116199895718838, "skew pk-pk"=1.5110834424588262, "skews"=[-74.69136893305789, -75.7530157737499, -74.24193233129107, -75.09692280821177, -75.74111325102723, -74.86974243975591, -74.71563006478846, -75.22775992262068, -74.35390192589017, -74.90218739687595]}, {"frequency (Hz)"=750000000.0, "mean skew"=-74.95763910484766, "skew std dev"=0.5677528933215689, "skew pk-pk"=2.123037675926298, "skews"=[-73.82145504629973, -75.94449272222603, -74.67944302979093, -75.33228944620532, -74.8932192302571, -74.49762145754268, -75.04957226562384, -74.85329596223187, -75.32159348100768, -75.1834084072915]}, {"frequency (Hz)"=800000000.0, "mean skew"=-75.1311015283594, "skew std dev"=0.33970208894817877, "skew pk-pk"=0.9989241671122215, "skews"=[-75.67452521283357, -74.68056519178819, -75.2691114789633, -74.85528455661031, -74.94487479500677, -75.38656756142882, -75.09206762893128, -74.67560104572135, -75.25292836967753, -75.47948944263278]}, {"frequency (Hz)"=850000000.0, "mean skew"=-75.26706597906876, "skew std dev"=0.6418642775263751, "skew pk-pk"=2.0484569340382137, "skews"=[-75.58806533849115, -74.73727713594762, -75.9789686940783, -75.55597935744332, -76.04301551609053, -75.20302665430759, -75.57132276741197, -74.63017769456576, -73.99455858205232, -75.36826805029901]}, {"frequency (Hz)"=900000000.0, "mean skew"=-74.65826036989716, "skew std dev"=0.7970046190553706, "skew pk-pk"=2.4181003309397653, "skews"=[-74.83136822856201, -73.89652167540036, -74.14121163043865, -75.27772774410819, -75.88029401046524, -73.86107333334851, -74.63915243708949, -75.09520441207107, -75.49785654796266, -73.46219367952547]}, {"frequency (Hz)"=950000000.0, "mean skew"=-74.88264264004111, "skew std dev"=0.5088708463887421, "skew pk-pk"=1.6771581841278334, "skews"=[-74.56204888426032, -74.84739680207673, -74.86975522653512, -75.57244373421409, -75.0619492890494, -74.33700452782378, -74.98864724396006, -75.39716203671183, -75.29473310569372, -73.89528555008626]}, {"frequency (Hz)"=1000000000.0, "mean skew"=-75.53121285044428, "skew std dev"=0.2736923101362065, "skew pk-pk"=0.799963574568821, "skews"=[-75.14141955835609, -75.92491368005396, -75.67661540694397, -75.81629629380201, -75.12495010548514, -75.6475063102048, -75.65590517618044, -75.461216790678, -75.58325733595903, -75.28004784677937]}] {"frequency (Hz)" format="%#_6p"; "mean skew" format="%#_6p"; "skew std dev" format="%#_6p"; "skew pk-pk" format="%#_6p"; "skews" format="%#_6p"}
  out "Current Frequency Under Test":dbl=1000000000.0 format="%#_6p"
  in  "DUC Freq Shift (Hz)":dbl=1000000000.0 format="%#_4p"
  in  "DDC Freq Shift (Hz)":dbl=1000000000.0 format="%#_4p"
  in  "IQ Enabled":bool=TRUE
  in  "DDC Enabled":bool=TRUE
  in  "processing mode":T2=enum."None, Two Channels"
  out "AO num Samples":i32=32
  in  "waveform config":T3(array[cluster])=[{"Frequency (Hz)"=0.0, "Amplitude (V)"=1.0, "Phase (Deg)"=0.0}, {"Frequency (Hz)"=0.0, "Amplitude (V)"=1.0, "Phase (Deg)"=0.0}] {"Phase (Deg)" format="%.2p"; "Amplitude (V)" format="%0.2p"; "Frequency (Hz)" format="%0.2p"}
  in  "reference clock source":T4 items=["Default", "Onboard", "PXI_Clk10", "External", "None", "Baseboard Reference"]
  in  "Update Waveform":bool caption="Download AO Waveforms"
  out "Sample Rate":dbl=1600000000.0 format="%#_6p"
  in  "ADC Interleaving Factor":i32=1 min=0 max=2 step=1
  in  "AI num samples":u64=1024 step=32
  in  "AI channels":string="AI0,AI1"
  out "Device Power":dbl(slide)=33.42 scale=-1.0..58.0 scale format="%#_3p"
  out "FPGA Temperature":dbl(slide)=50.0 scale=0.0..100.0 scale format="%#_3p"
  in  "Trigger Type":enum32{"Immediate", "Analog", "Digital"}(tab)
  in  "trigger channel":string="AI0"
  in  "rising edge?":bool=TRUE
  in  "level (V)":dbl format="%#_3p"
  in  "hysteresis (V)":dbl=0.01 format="%#_3p"
  in  "digital trigger source":string(combo)
  in  "stop":bool
  in  "Bitfile path":path=path "C:/Repos/bsherman-sandbox/CogRF/5785 Measurements/Common/Original 5785 Example/FPGA Bitfiles/PXIe_5785_KU060.lvbitx"
  in  "Waveform Tab Control":T5(tab)=enum."AO Generated Waveform"
  out "Waveform Graph":waveform(dbl)[](graph)=[{"t0"=timestamp(0 s since 1904-01-01), "dt"=6.25e-10, "Y"=array[1024 elements]}, {"t0"=timestamp(0 s since 1904-01-01), "dt"=6.25e-10, "Y"=array[1024 elements]}, {"t0"=timestamp(0 s since 1904-01-01), "dt"=6.25e-10, "Y"=array[1024 elements]}, {"t0"=timestamp(0 s since 1904-01-01), "dt"=6.25e-10, "Y"=array[1024 elements]}]
  out "FFT":cluster{"f0":dbl, "df":dbl, "magnitude":dbl[]}[](graph)=[{"f0"=0.0, "df"=1562500.0, "magnitude"=[-77.13572579029565, -80.45708666326453, -103.79245112843186, -97.98137656824686, -94.57200722176353, -92.65763152377897, -95.98726843937527, -102.86795010945991, -96.14954496799203, -94.67889969508705, -105.32880703411237, -109.75338541511155, -98.45052236962857, -99.97277928897853, -97.67341689514296, -96.55942931040256, -96.63934380086813, -107.64381725733759, -102.84951934545217, -97.01870899638665, -92.78292767025631, -92.55128163694627, -99.80050165821275, -100.14449129437551, -98.70128185500639, -102.55067663406187, -97.39101705964808, -91.83266790730308, -90.75650181516296, -98.64712922168314, -106.17088277221767, -96.34516841804978, -100.89392344803926, -99.78325798079545, -102.50405947434437, -92.38929201729701, -91.56845242496799, -103.75158542276148, -99.52351384372717, -98.42337697765277, -93.70487312349073, -91.52417894943171, -95.2756436991707, -96.89764886053568, -95.4757035963045, -100.2922929330799, -97.30882426543579, -91.39987545891105, -94.33957625033418, -98.64884295864542, -97.68681355030056, -97.15412038044867, -108.12739544631653, -98.28060292686587, -98.45371129063521, -101.51021754359725, -98.76754647693897, -100.08185584703925, -113.0590073458177, -100.68870367947974, -102.92557436557672, -96.29657591290183, -99.03366216745607, -95.1174080182553, -94.67585787301235, -100.34149556769964, -103.1395692383062, -101.3744844011393, -97.25073703452382, -99.11844816850896, -94.74885649893407, -97.21473681755967, -98.84560268994497, -95.57423097988257, -105.42901715309334, -94.8797122859792, -94.76816250532164, -99.63546732313955, -95.47162304037047, -97.40982480106781, -103.04255633829905, -101.65227459783648, -99.07491754899341, -105.72237245393504, -98.06751631068069, -103.82696091330175, -106.52337890502727, -94.70253204241224, -91.39001704432003, -95.4209099902308, -106.41074807396441, -106.67560785995136, -106.99264436321884, -101.62701756112224, -102.25421114796886, -110.50921527442716, -107.82878561446813, -115.38298754096292, -97.37279608863462, -104.43888113188648, -107.69721574819135, -97.37083951410577, -98.00658387662654, -98.50955456344397, -94.71891192794091, -104.30244036433784, -93.10518434698493, -89.4661009169698, -93.82425515605544, -97.14395908708623, -92.89810051564768, -95.43869909750379, -103.78566181845298, -99.80902352162643, -104.57055589085145, -97.74795969915886, -96.71654435580754, -97.68158991538297, -98.74136093054881, -104.43115431403827, -96.05961346555027, -97.95262224589486, -101.42210652922181, -100.02819790398229, -95.55436090423443, -97.57728407319306, -100.90626757862498, -93.31236177109437, -91.272421318652, -95.30404811613268, -103.12492265039724, -93.35676944154777, -94.00526629104151, -102.28046695005395, -106.53764411629687, -107.56279761831236, -101.5593634925766, -98.2141207382466, -94.02296254528582, -96.53399084093948, -98.94959879275405, -93.42823287335882, -94.94951574706883, -97.08874623358447, -105.03146680674698, -98.75309433013088, -109.1695415196823, -105.59976779527558, -107.76013052471781, -102.82849666261647, -97.52659005579636, -106.83879824373705, -96.10942823239937, -96.65230592383325, -100.67929749170221, -104.06634915757894, -111.70088808039834, -97.2813289607887, -94.83113615835136, -92.9141490183961, -94.22400861219059, -97.10847074440795, -96.6466729718128, -95.79585849359775, -97.6526507483648, -98.42774407401663, -101.8670300153706, -93.86649098375386, -91.0966271580726, -91.51616642750085, -103.14115641130826, -91.6241821720606, -92.40820093306878, -92.04652228935632, -102.33801946688314, -95.51353629387735, -95.99100291351647, -100.4023102259629, -95.28557402678535, -94.5504496911188, -96.74258260232651, -106.1385148983767, -95.91299009352633, -94.7451401086726, -106.27679463206957, -95.66355412978544, -96.89611735038073, -106.49564436592962, -104.39849413750247, -99.79993222438658, -107.27578024108954, -99.94892477964382, -91.64740708301525, -90.32708979865399, -92.63950017161781, -93.46483340712707, -92.52185739053986, -97.5507435661592, -101.40997990294954, -100.52826794191262, -93.8419358045948, -87.74050919691904, -86.17816433217571, -92.32208390318138, -110.83378944907425, -107.88640770845868, -98.73133711717303, -91.98490222122118, -93.11670505353862, -98.85061840926971, -90.05985533010175, -92.27241592387243, -106.33474473234101, -96.5105011259497, -97.50391394392318, -102.31517618422929, -100.46017932547272, -102.31393329125551, -102.07988555732362, -107.21039687170715, -105.58767866413905, -102.05881518831202, -100.86298907916051, -95.40350996033112, -91.16746108577794, -94.09243815374433, -97.65192666564448, -104.24944060126977, -101.082198157214, -94.4921647499718, -94.41243855332992, -98.21222259624678, -105.26142344954073, -94.28187223340848, -94.65714012057103, -91.9915249053831, -94.9860657180956, -100.57428942620186, -104.79327043871139, -98.39175590304123, -100.59990625433265, -101.58988888991726, -99.29117689490063, -102.03639787411022, -95.81212309648143, -98.0155095437292, -93.60506575713006, -94.02272699184182, -95.58388536061898, -96.77333458322101, -101.946975230775, -95.71429606054225, -102.58509231584397, -98.97382874032846, -96.57683507860533, -96.6010928083257, -94.71803434795501, -92.67476525519322, -93.68939051122794, -93.51749658846913, -96.40130225479945, -97.56084658528275, -97.15959577758782, -104.21758951863512, -93.11455331312457, -90.60030708653842, -92.6155641411707, -92.28572412377396, -93.68454451407555, -97.59487570579827, -95.06851083531691, -101.11972239269271, -99.53734019778331, -98.59303851330075, -96.29946678885304, -97.52463853183747, -114.7919489610357, -106.22356124792587, -98.21111002361451, -103.26697025273958, -101.19152690603988, -101.48653618573832, -97.60193847181661, -97.1017993461532, -102.00205074815393, -99.40568302792994, -103.1992032557979, -103.42488073024752, -100.51317880863814, -96.63608666705497, -96.49824466943174, -103.78580439432875, -108.7994024948285, -99.66333753741495, -100.50201652235802, -101.24382233932089, -101.72043908043963, -102.70464743313447, -108.48684113589478, -98.45082740431685, -95.98227240849852, -96.06614565788881, -100.42758574118012, -113.95537305155128, -102.70841841179578, -97.3006594757611, -93.66267228759442, -97.40878208802917, -106.42904562364839, -96.15914316335227, -91.5946048958632, -91.95775443139546, -94.56337477694339, -100.13978397205732, -95.07338737497321, -98.2950728098547, -110.77105465516043, -104.59548361598705, -97.61991306843903, -106.20422836047933, -100.88824471731664, -104.2092141704326, -100.01884639869729, -99.72896378603268, -107.13821882781167, -98.32238555156661, -103.08679138347617, -98.90309321138467, -93.40590701752787, -93.88984861747433, -103.27047406753013, -99.48664380170293, -96.0632145814715, -98.21452764716278, -103.13505117233234, -100.24831669353135, -99.34500743653275, -97.86855804766957, -96.3889708985043, -97.1822665656955, -93.8557844565402, -92.92614948966977, -93.63574598224199, -97.94382098708134, -107.16091825878655, -95.66774142831247, -97.15785484622437, -101.36184153102559, -99.84783835976977, -98.56553251712259, -107.54670002056982, -99.6829810184204, -96.36877546618464, -99.7744026403756, -100.87474752776438, -107.48225033897933, -96.32024229082852, -106.54990685920467, -104.25529459133963, -103.67147280138065, -98.29790399480868, -95.34135605233827, -93.59295941321048, -92.75619096183141, -95.73773925783317, -97.68491812754577, -104.68824180974343, -96.72027650133336, -93.79740736516958, -99.67470087284806, -102.48844324094512, -119.33849668958004, -97.95311305637335, -98.03290845451349, -109.92813968600555, -98.07615309602375, -106.52616781555051, -99.6849751911538, -96.64425644990203, -98.59308112139571, -91.25815887176316, -92.63942382696045, -107.30972823386031, -88.513427426363, -82.57143299337528, -86.07832263689247, -97.76813244665388, -96.85053373151122, -92.45310141321727, -97.47188117918495, -99.42909730421889, -99.66576945172314, -96.73234360821432, -93.85678530537555, -99.71086252140283, -106.1084368814814, -95.67291094471057, -99.91727626021957, -112.30689570310818, -99.76608494187865, -99.90037720021579, -101.42249194247283, -94.56835175002814, -91.55315452210402, -93.1071095119886, -92.88617147761198, -93.41410142699797, -95.09099701452425, -95.4498114817717, -93.16377976922672, -90.80316127838627, -92.3282321234731, -93.69355230753104, -97.08306849558335, -109.25102287908948, -101.78727612337055, -106.16666766319996, -97.30752647860312, -93.80564977139943, -115.84900494976497, -94.93097728996334, -105.16123231517122, -97.99402723034086, -98.85487400446047, -108.10868832806207, -96.63566126201482, -102.92959112396188, -109.64230379478659, -107.81563351436873, -110.37807325697962, -101.02537677819006, -100.57269348096986, -107.05022642658261, -95.24908039362768, -94.22712464498402, -100.16100602454318, -90.57445452117517, -89.89797914734568, -97.01549039588502, -111.45359537452366, -102.0432416346108, -104.35545719932222, -110.4183041068236, -105.85784695396345, -105.57751118767132, -105.45720711768513, -106.71799635104057, -95.18082018381199, -92.41803688928456, -92.5980608827961, -92.84681028238558, -93.23162058885329, -96.5136752902513, -100.94373704283183, -98.03654927679065, -100.01852988802234, -102.41929595068596, -103.9799144598686, -104.96197412910433, -98.55473132166813, -97.44987670874485, -98.61008815312161, -114.05794270099929, -98.85678715631323, -99.6300056399385, -104.7821521725495, -93.88577414959576, -97.93243717134494, -100.94313705727082, -95.18081832568022, -101.72271880559911, -104.70004943063029, -105.16436436799644, -103.50959519496784, -101.75802952651956, -96.52115443190384, -96.10402967503681, -104.42948547009789, -94.34472607647314, -96.92108915454432, -96.0606453749378, -98.79979736665932, -91.31398241357729, -95.990363923125, -96.0343550440477, -92.23393269940125, -108.22586678084357, -94.79767697255843, -96.47790619945093, -102.1641876124531, -105.68843543623451, -104.1330435212331, -100.91286718710485, -96.33731257457063, -95.14290078297103, -93.57630380674406, -91.1549450437296, -93.76176898982386, -100.73077574965858, -101.84911089736966, -100.9021334676966, -106.68216565424879, -98.7285849211363, -98.54015639653579, -95.31939044064701, -93.81179846374295, -97.09331825398627, -93.92095769831582, -104.83830680764831, -93.58337248389418, -93.72865626020084, -101.29309635727355]}, ...(4 in all)] caption="Waveform Graph"
  out "detected frequencies":dbl[](array[numeric])=[1000003554.6699688, 1000002325.6067231] format="%_4p"
  out "AO Out":waveform(dbl)[](graph)=[{"t0"=timestamp(0 s since 1904-01-01), "dt"=1.0, "Y"=[1.0, 1.0, 1.0, 1.0, 1.0, 1.0, 1.0, 1.0, 1.0, 1.0, 1.0, 1.0, 1.0, 1.0, 1.0, 1.0, 1.0, 1.0, 1.0, 1.0, 1.0, 1.0, 1.0, 1.0, 1.0, 1.0, 1.0, 1.0, 1.0, 1.0, 1.0, 1.0]}, {"t0"=timestamp(0 s since 1904-01-01), "dt"=1.0, "Y"=[1.0, 1.0, 1.0, 1.0, 1.0, 1.0, 1.0, 1.0, 1.0, 1.0, 1.0, 1.0, 1.0, 1.0, 1.0, 1.0, 1.0, 1.0, 1.0, 1.0, 1.0, 1.0, 1.0, 1.0, 1.0, 1.0, 1.0, 1.0, 1.0, 1.0, 1.0, 1.0]}] caption="Waveform Graph"
  out "Limit (W)":dbl=58.0
  out "Power (W)":dbl=33.42
  out "Limit (C)":dbl=96.0
  out "Temp (C)":dbl=50.0 format="%#_4p"
  in  "RIO Device":T6="5785_00"
  # "Resource Configuration"
  # "Clocking configuration"
  # "Input Waveform Configuration"
  # "Device Monitoring"
  # "Output Waveform Configuration"
  # "Digital Upconverter Configuration"
  # "Frequency (Hz)"
  # "Amplitude (V)"
  # "Phase (Deg)"
  # "AO 0"
  # "AO 1"
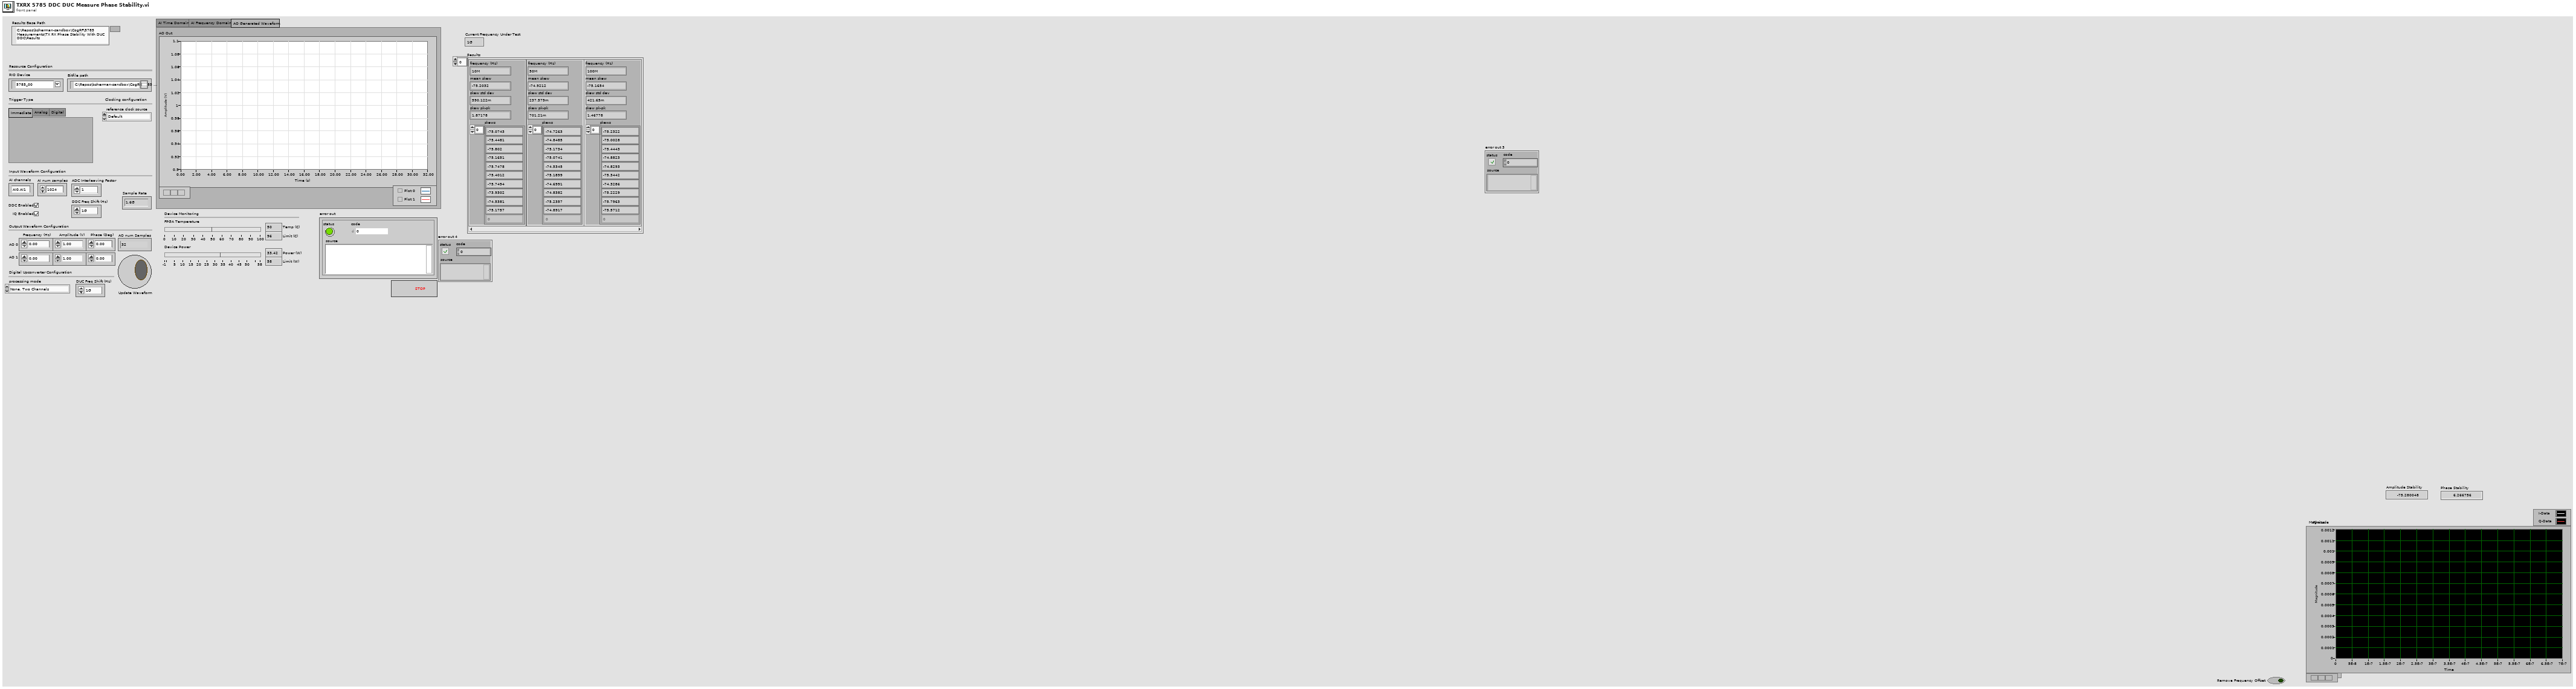
[diagram p1: front panel]
types:
  T1 = cluster{"frequency (Hz)":dbl, "mean skew":dbl, "skew std dev":dbl, "skew pk-pk":dbl, "skews":dbl[]}[]
  T2 = typedef "GettingStarted_5785_Host.lvlib/Upconversion Mode.ctl" = enum16{"None, One Channel", "None, Two Channels", "FPGA-only, One Channel", "DAC and FPGA, One Channel", "DAC-only, One Channel"}
  T3 = cluster{"Frequency (Hz)":dbl, "Amplitude (V)":dbl, "Phase (Deg)":dbl}[]
  T4 = typedef "NI FlexRIO API v1.lvlib/Reference Clock Source.ctl" = i32
  T5 = enum32{"AI Time Domain", "AI Frequency Domain", "AO Generated Waveform"}
  T6 = typedef "nirio_resource_slv.ctl" = tag
  T7 = cluster{"averaging mode":enum16{"No averaging", "Vector averaging", "RMS averaging", "Peak hold"}, "weighting mode":enum16{"Linear", "Exponential"}, "number of averages":u32}
  T8 = cluster{"frequency":dbl, "mean skew":dbl, "skew std dev":dbl, "skew pk-pk":dbl, "skews":dbl[]}
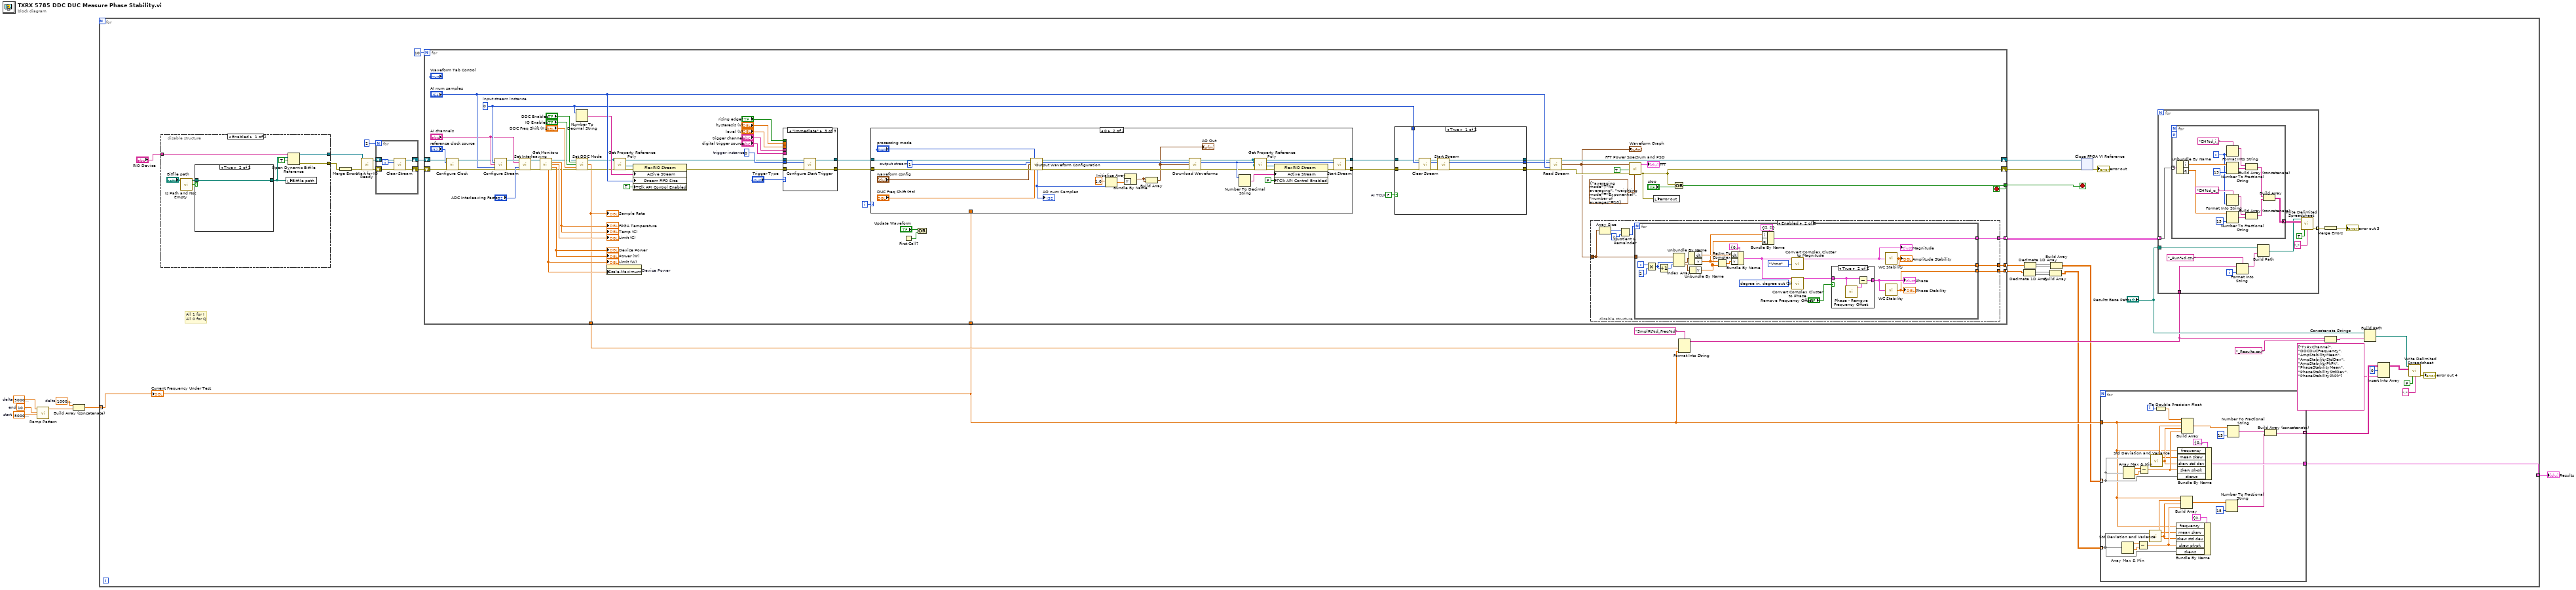
[diagram p0: block diagram]
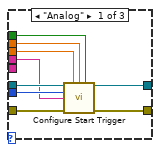
[diagram p3: hidden frame]
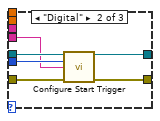
[diagram p4: hidden frame]
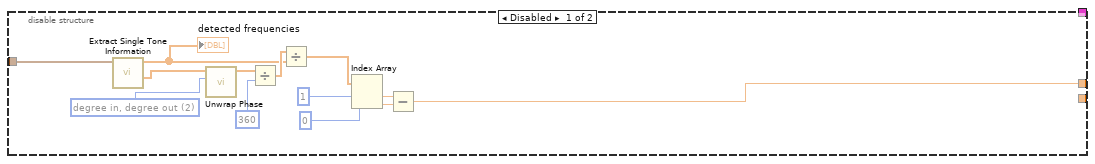
[diagram p5: hidden frame]
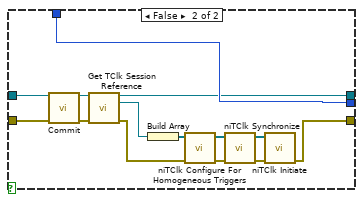
[diagram p7: hidden frame]
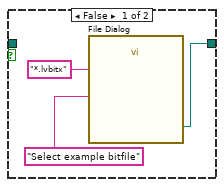
[diagram p8: hidden frame]
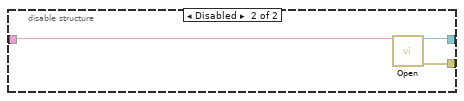
[diagram p9: hidden frame]
diagram:
  w4 = 10000000.0  # delta
  w5 = 50000000.0  # delta
  w6 = 1000000000.0  # end
  w7 = 50000000.0  # start
  n1 = call-poly <vilib>:"Ramp Pattern.vi"("start"=w7, "end"=w6, "delta"=w5) -> ("Ramp Pattern"=w1:dbl[])  [unwired: 6 in, 2 out]
  n2 = Build Array (concatenate)(w4, w1) -> (w2:dbl[])
  n3 = for {
    tunnel: [w36] -> w3 mode=indexing
    tunnel: w2 -> [w19] mode=indexing
    stop <- w37 stop-if-true
    # "All 1 for I\nAll 0 for Q"
    n4 = disable-structure shown="Enabled" {
      disable-tunnel: [w288 w295] -> w48
      disable-tunnel: [w287 w294] -> w47
      disable-tunnel: "RIO Device" -> [w286 w293]
      frame Enabled {
        n5 = call <vilib>:"Is Path and Not Empty.vi"("path"="Bitfile path") -> ("Is Path and Not Empty?"=w283:bool)  [unwired: 4 in]
        n6 = case shown="True" w283 {
          tunnel: "Bitfile path" -> [_ w292]
          tunnel: [w290 w292] -> w282
          frame False {
            n7 = call "File Dialog"("prompt"="Select example bitfile", "pattern (all files)"="*.lvbitx") -> ("selected path"=w290:path)  [unwired: 10 in, 3 out]
          }
          frame True {
          }
        }
        n8 = local write "Bitfile path"(w282) -> ()
        n9 = Open Dynamic Bitfile Reference(0:w286, 1:w282, 2:TRUE ("Run When Loaded")) -> (5:w287:refnum<k20>, 8:w288:errorcluster)  [unwired: 2 in]
      }
      frame Disabled {
        n10 = call <instrlib>:"Open.vi"("RIO Device"=w293) -> ("fpga interface out"=w294:refnum<k20>, "error out"=w295:errorcluster)  [unwired: 13 in]
      }
    }
    n11 = Merge Errors(w48) -> (w35:errorcluster)
    n12 = call <instrlib>:"Wait for IO Ready.vi"("fpga interface in"=w47, "error in"=w35) -> ("fpga interface out"=w43:refnum<k20>, "error out"=w42:errorcluster)  [unwired: 10 in, 2 out]
    n13 = for {
      N: 2 -> [_]
      shift-right: [w227] -> w40
      shift-left: w43 -> [w230]
      shift-right: [w228] -> w41
      shift-left: w42 -> [w229]
      i -> [w226]
      n14 = call <instrlib>:"Clear Stream.vi"("fpga interface in"=w230, "stream instance"=w226, "error in"=w229) -> ("fpga interface out"=w227:refnum<k20>, "error out"=w228:errorcluster)  [unwired: 10 in, 1 out]
    }
    n15 = for {
      N: 10 -> [_]
      shift-right: [w74] -> w44
      shift-left: w41 -> [w109]
      shift-right: [w107] -> w45
      shift-left: w40 -> [w108]
      tunnel: [w58] -> w37
      tunnel: [w57] -> w13 mode=concatenating
      tunnel: w19 -> [w56]
      tunnel: [w53] -> w32
      tunnel: [w50] -> w20 mode=indexing
      tunnel: [w49] -> w10 mode=concatenating
      i -> [w52]
      stop <- w58 stop-if-true
      w54 = FALSE  # AI TCLK
      w98 = u32 0  # trigger instance
      w94 = u32 0  # input stream instance
      n16 = call-poly <instrlib>:"Configure Clock.vi"("fpga interface in"=w108, "reference clock source"="reference clock source", "error in"=w109) -> ("fpga interface out"=w76:refnum<k20>, "error out"=w102:errorcluster)  [unwired: 11 in]
      n17 = call <instrlib>:"Configure Stream.vi"("fpga interface in"=w76, "stream instance"=w94, "channels enabled"="AI channels", "num samples"="AI num samples", "error in"=w102) -> ("fpga interface out"=w92:refnum<k20>, "error out"=w90:errorcluster)  [unwired: 7 in, 2 out]
      n18 = call "Set Interleaving.vi"("fpga interface in"=w92, "AI channels enabled"="AI channels", "ADC Interleaving Factor"="ADC Interleaving Factor", "error in (no error)"=w90) -> ("fpga interface out"=w78:refnum<k20>, "error out"=w77:errorcluster)  [unwired: 10 in]
      n19 = call "Get Monitors.vi"("fpga interface in"=w78, "error in (no error)"=w77) -> ("fpga interface out"=w66:refnum<k20>, "FPGA Temperature (C)"=→"Temp (C)" →"FPGA Temperature":dbl, "Temperature Limit (C)"=→"Limit (C)":dbl, "Total Power (W)"=→"Power (W)" →"Device Power":dbl, "Power Limit (W)"=w84:dbl, "error out"=w65:errorcluster)  [unwired: 8 in]
      "Limit (W)" <- w84
      n20 = Number To Decimal String(number=w94) -> (decimal integer string=w100:string)  [unwired: 1 in]
      n21 = call "Set DDC Mode.vi"("fpga refnum"=w66, "DDC Enabled"="DDC Enabled", "IQ Enabled"="IQ Enabled", "DDC Frequency Shift (Hz)"="DDC Freq Shift (Hz)", "error in (no error)"=w65) -> ("fpga refnum out"=w67:refnum<k20>, "sample rate"=w53:dbl, "error out"=w68:errorcluster)  [unwired: 8 in]
      "Sample Rate" <- w53
      n22 = property on="Device Power" class="Slide (strict)"("Scale.Maximum"=w84) -> ()  [unwired: 2 in, 2 out]
      n23 = call-poly <instrlib>:"Get Property Reference Poly.vi"("error in (no error)"=w68, "fpga interface in"=w67) -> ("error out"=w89:errorcluster, "property reference"=w88:refnum<k20>)  [unwired: 4 in, 1 out]
      n24 = property class="FlexRIO Stream"(reference=w88, error in=w89, "Active Stream"=w100, "Stream FIFO Size"="AI num samples", "TClk API Control Enabled"=TRUE ("Configuration:TClk API Control Enabled")) -> (error out=w97:errorcluster)  [unwired: 1 out]
      n25 = case shown="\"Immediate\"" "Trigger Type" {
        tunnel: w67 -> [w144 w150 w155]
        tunnel: w97 -> [w143 w149 w154]
        tunnel: [w142 w148 w153] -> w96
        tunnel: [w141 w147 w152] -> w95
        tunnel: w98 -> [w140 w146 w151]
        tunnel: "trigger channel" -> [w139 _ _]
        tunnel: "level (V)" -> [w138 _ _]
        tunnel: "hysteresis (V)" -> [w137 _ _]
        tunnel: "rising edge?" -> [w136 _ _]
        tunnel: "digital trigger source" -> [_ w145 _]
        frame "Analog" {
          n26 = call-poly <instrlib>:"Configure Start Trigger.vi"("fpga interface in"=w144, "level"=w138, "hysteresis"=w137, "rising edge?"=w136, "trigger instance"=w140, "channel"=w139, "error in"=w143) -> ("fpga interface out"=w142:refnum<k20>, "error out"=w141:errorcluster)  [unwired: 6 in, 1 out]
        }
        frame "Digital" {
          n27 = call-poly <instrlib>:"Configure Start Trigger.vi"("fpga interface in"=w150, "trigger instance"=w146, "trigger source"=w145, "error in"=w149) -> ("fpga interface out"=w148:refnum<k20>, "error out"=w147:errorcluster)  [unwired: 9 in, 1 out]
        }
        frame "Immediate" {
          n28 = call-poly <instrlib>:"Configure Start Trigger.vi"("fpga interface in"=w155, "trigger instance"=w151, "error in"=w154) -> ("fpga interface out"=w153:refnum<k20>, "error out"=w152:errorcluster)  [unwired: 10 in, 1 out]
        }
      }
      n29 = case shown="0" w52 {
        tunnel: [w111 w135] -> w73
        tunnel: [w110 w134] -> w72
        tunnel: w96 -> [w111 w133]
        tunnel: w95 -> [w110 w132]
        tunnel: w56 -> [_ _]
        frame 1.., Default {
        }
        frame 0 {
          w131 = u32 1  # output stream
          n30 = call "Output Waveform Configuration.vi"("Refnum in"=w133, "processing mode"="processing mode", "output stream instance"=w131, "waveform config"="waveform config", "error in (no error)"=w132, "DUC Frequency Shift"="DUC Freq Shift (Hz)") -> ("Refnum out"=w122:refnum<k20>, "output stream instance out"=w121:u32, "ao wfm samples"=w116:i32, "error out"=w118:errorcluster)  [unwired: 5 in, 1 out]
          "AO num Samples" <- w116
          n31 = Initialize Array(1.0 ("element"), w116) -> (w114:dbl[])
          n32 = Bundle By Name("Y"=w114) -> (w112:waveform(dbl))  [unwired: 1 in]
          n33 = Build Array(w112, w112) -> (w113:waveform(dbl)[])
          "AO Out" <- w113
          n34 = call "Download Waveforms.vi"("fpga interface in"=w122, "stream instance"=w121, "waveforms"=w113, "error in"=w118) -> ("fpga interface out"=w119:refnum<k20>, "stream instance out"=w120:u32, "error out"=w117:errorcluster)  [unwired: 9 in]
          n35 = Number To Decimal String(number=w120) -> (decimal integer string=w123:string)  [unwired: 1 in]
          n36 = call-poly <instrlib>:"Get Property Reference Poly.vi"("error in (no error)"=w117, "fpga interface in"=w119) -> ("error out"=w127:errorcluster, "property reference"=w126:refnum<k20>)  [unwired: 4 in, 1 out]
          n37 = property class="FlexRIO Stream"(reference=w126, error in=w127, "Active Stream"=w123, "TClk API Control Enabled"=FALSE ("Configuration:TClk API Control Enabled")) -> (error out=w124:errorcluster)  [unwired: 1 out]
          n38 = call <instrlib>:"Start Stream.vi"("fpga interface in"=w119, "stream instance"=w120, "error in"=w124) -> ("fpga interface out"=w135:refnum<k20>, "error out"=w134:errorcluster)  [unwired: 10 in, 1 out]
        }
      }
      n39 = First Call?() -> (First Call?: T/F=w63:bool)
      n40 = Or(x="Update Waveform", y=w63) -> ()  [unwired: 1 out]
      n41 = case shown="True" w54 {
        tunnel: w94 -> [w211 w223]
        tunnel: w73 -> [w210 w225]
        tunnel: w72 -> [w209 w224]
        tunnel: [w208 w223] -> w62
        tunnel: [w207 w222] -> w61
        tunnel: [w206 w221] -> w60
        frame True {
          n42 = call <instrlib>:"Clear Stream.vi"("fpga interface in"=w210, "stream instance"=w211, "error in"=w209) -> ("fpga interface out"=w205:refnum<k20>, "stream instance out"=w204:u32, "error out"=w203:errorcluster)  [unwired: 10 in]
          n43 = call <instrlib>:"Start Stream.vi"("fpga interface in"=w205, "stream instance"=w204, "error in"=w203) -> ("fpga interface out"=w207:refnum<k20>, "stream instance out"=w208:u32, "error out"=w206:errorcluster)  [unwired: 10 in]
        }
        frame False {
          n44 = call <instrlib>:"Commit.vi"("fpga interface in"=w225, "error in"=w224) -> ("fpga interface out"=w220:refnum<k20>, "error out"=w219:errorcluster)  [unwired: 12 in]
          n45 = call <instrlib>:"Get TClk Session Reference.vi"("fpga interface in"=w220, "error in"=w219) -> ("fpga interface out"=w222:refnum<k20>, "tclk session reference"=w217:refnum<k20>, "error out"=w218:errorcluster)  [unwired: 11 in]
          n46 = Build Array(w217) -> (w216:refnum<k20>[])
          n47 = call <instrlib>:"niTClk Configure For Homogeneous Triggers.vi"("error in (no error)"=w218, "sessions"=w216) -> ("error out"=w214:errorcluster, "sessions out"=w215:refnum<k20>[])  [unwired: 8 in]
          n48 = call <instrlib>:"niTClk Synchronize.vi"("error in (no error)"=w214, "sessions"=w215) -> ("error out"=w212:errorcluster, "sessions out"=w213:refnum<k20>[])  [unwired: 8 in]
          n49 = call <instrlib>:"niTClk Initiate.vi"("error in (no error)"=w212, "sessions"=w213) -> ("error out"=w221:errorcluster)  [unwired: 8 in, 1 out]
        }
      }
      n50 = call-poly <instrlib>:"Read Stream.vi"("fpga interface in"=w61, "stream instance"=w62, "samples"="AI num samples", "error in"=w60) -> ("fpga interface out"=w107:refnum<k20>, "read data"=w51:waveform(dbl)[], "error out"=w80:errorcluster)  [unwired: 7 in, 2 out]
      "Waveform Graph" <- w51
      n51 = disable-structure shown="Enabled" {
        disable-tunnel: [w157 w170] -> w57
        disable-tunnel: w51 -> [w156 w175]
        disable-tunnel: [_ w171] -> w50
        disable-tunnel: [_ w169] -> w49
        frame Disabled {
          w164 = 2 items=["radian in, radian out", "radian in, degree out", "degree in, degree out", "degree in, radian out"] ("phase unit")
          n52 = call-poly <vilib>:"Extract Single Tone Information.vi"("time signals in"=w156) -> ("detected phases (deg)"=w163:dbl[], "detected frequencies"=w158:dbl[])  [unwired: 5 in, 4 out]
          "detected frequencies" <- w158
          n53 = call <vilib>:"Unwrap Phase.vi"("phase unit"=w164, "Phase"=w163) -> ("Unwrapped Phase"=w168:dbl[])  [unwired: 8 in, 1 out]
          n54 = Divide(x=w168, y=360) -> (x/y=w167:dbl[])
          n55 = Divide(x=w167, y=w158) -> (x/y=w165:dbl[])
          n56 = Index Array(array=w165, index #1=1 ("index (row)"), index #2=0 ("index (row)")) -> (element #1=w160:dbl, element #2=w159:dbl)
          n57 = Subtract(x=w160, y=w159) -> (x-y=w157:dbl)
        }
        frame Enabled {
          n58 = Array Size(array=w175) -> (size(s)=w174:i32)
          n59 = Quotient & Remainder(x=w174, y=2) -> (floor(x/y)=w172:i32)  [unwired: 1 out]
          n60 = for {
            N: w172 -> [_]
            tunnel: w175 -> [w198]
            tunnel: [w181] -> w170 mode=indexing
            tunnel: [w180] -> w169 mode=indexing
            tunnel: [w176] -> w171 mode=indexing
            i -> [w197]
            w187 = 2 items=["radian in, radian out", "radian in, degree out", "degree in, degree out", "degree in, radian out"] ("phase unit")
            n61 = Multiply(x=w197, y=2) -> (x*y=w195:i32)
            n62 = Increment(x=w195) -> (x+1=w194:i32)
            n63 = Index Array(array=w198, index #1=w195, index #2=w194) -> (element #1=w193:waveform(dbl), element #2=w192:waveform(dbl))
            n64 = Unbundle By Name(w193) -> ("dt"=w190:dbl, "Y"=w179:dbl[])
            n65 = Unbundle By Name(w192) -> ("Y"=w178:dbl[])
            n66 = Re/Im To Complex(1:w178, 2:w179) -> (0:w189:cdb[])
            n67 = Bundle By Name(cluster=cluster{"t0":dbl, "dt":dbl, "Y":cdb[]} {"t0"=0.0, "dt"=0.0, "Y"=[]} ("RX Sample Rate: 1MSps 2"), "dt"=w190, "Y"=w189) -> (w182:cluster{"t0":dbl, "dt":dbl, "Y":cdb[]})
            n68 = Bundle By Name(cluster=cluster{"i":dbl[], "q":dbl[]} {"i"=[], "q"=[]}, "i"=w179, "q"=w178) -> (w176:cluster{"i":dbl[], "q":dbl[]})
            n69 = call "Convert Complex Cluster to Magnitude.vi"("IQ data (complex) In"=w182, "Public.Units"=enum8{"Vrms", "dBm"}."Vrms") -> ("Magnitude Out"=w184:cluster{"t0":dbl, "dt":dbl, "Y":dbl[]})  [unwired: 12 in, 1 out]
            "Magnitude" <- w184
            n70 = call "Convert Complex Cluster to Phase.vi"("IQ data (complex) In"=w182, "phase unit"=w187) -> ("Phase Out"=w186:cluster{"t0":dbl, "dt":dbl, "Y":dbl[]})  [unwired: 12 in, 1 out]
            n71 = case shown="True" "Remove Frequency Offset" {
              tunnel: w186 -> [w199 w201]
              tunnel: [w199 w200] -> w183
              frame False {
              }
              frame True {
                n72 = call "Phase - Remove Frequency Offset.vi"("Phase In"=w201) -> ("Phase Out"=w202:cluster{"t0":dbl, "dt":dbl, "Y":dbl[]})  [unwired: 13 in, 1 out]
                n73 = Subtract(x=w201, y=w202) -> (x-y=w200:cluster{"t0":dbl, "dt":dbl, "Y":dbl[]})
              }
            }
            "Phase" <- w183
            n74 = call "WC Stability.vi"("Data In"=w184) -> ("Stability"=w181:dbl)  [unwired: 4 in]
            "Amplitude Stability" <- w181
            n75 = call "WC Stability.vi"("Data In"=w183) -> ("Stability"=w180:dbl)  [unwired: 4 in]
            "Phase Stability" <- w180
          }
        }
      }
      n76 = call-poly <vilib>:"FFT Power Spectrum and PSD.vi"("averaging parameters"=T7 {"averaging mode"=enum."No averaging", "weighting mode"=enum."Exponential", "number of averages"=10}, "error in (no error)"=w80, "dB On (F)"=TRUE, "time signals"=w51) -> ("error out"=w74:errorcluster, "Power Spectrum / PSD"=→"FFT":cluster{"f0":dbl, "df":dbl, "magnitude":dbl[]}[])  [unwired: 4 in, 2 out]
      n77 = local write "error out"(w74) -> ()
      n78 = Or(x=w74, y="stop") -> (x .or. y?=w58:bool)
    }
    n79 = Format Into String(format string="SmplRt%d_Freq%d", w32, w19) -> (resulting string=w22:string)  [unwired: 2 in, 1 out]
    n80 = Decimate 1D Array(w10) -> (w11:dbl[], w8:dbl[])
    n81 = Decimate 1D Array(w13) -> (w15:dbl[], w14:dbl[])
    n82 = Build Array(w11, w8) -> (w9:dbl[][])
    n83 = Build Array(w15, w14) -> (w12:dbl[][])
    n84 = xnode "Close FPGA VI Reference"("FPGA VI Reference In"=w45, "error in"=w44) -> ("error out"=→"error out":errorcluster)
    n85 = for {
      tunnel: [w255] -> w36
      tunnel: w12 -> [w254] mode=indexing
      tunnel: w19 -> [w236]
      tunnel: [w231] -> w18 mode=indexing
      tunnel: w9 -> [w237] mode=indexing
      i -> [w235]
      n86 = Array Max & Min(array=w237) -> (max value=w242:dbl, min value=w241:dbl)  [unwired: 2 out]
      n87 = Array Max & Min(array=w254) -> (max value=w250:dbl, min value=w249:dbl)  [unwired: 2 out]
      n88 = Subtract(x=w242, y=w241) -> (x-y=w245:dbl)
      n89 = Subtract(x=w250, y=w249) -> (x-y=w253:dbl)
      n90 = call <vilib>:"Std Deviation and Variance.vi"("X"=w237) -> ("mean"=w243:dbl, "standard deviation"=w244:dbl)  [unwired: 1 in, 1 out]
      n91 = call <vilib>:"Std Deviation and Variance.vi"("X"=w254) -> ("mean"=w251:dbl, "standard deviation"=w252:dbl)  [unwired: 1 in, 1 out]
      n92 = To Double Precision Float(number=w235) -> (double precision float=w234:dbl)
      n93 = Bundle By Name(cluster=T8 {"frequency"=0.0, "mean skew"=0.0, "skew std dev"=0.0, "skew pk-pk"=0.0, "skews"=[]}, "frequency"=w236, "mean skew"=w243, "skew std dev"=w244, "skew pk-pk"=w245, "skews"=w237) -> ()  [unwired: 1 out]
      n94 = Bundle By Name(cluster=T8 {"frequency"=0.0, "mean skew"=0.0, "skew std dev"=0.0, "skew pk-pk"=0.0, "skews"=[]}, "frequency"=w236, "mean skew"=w251, "skew std dev"=w252, "skew pk-pk"=w253, "skews"=w254) -> (w255:T8)
      n95 = Build Array(w236, w243, w244, w245) -> (w238:dbl[])
      n96 = Build Array(w234, w236, w251, w252, w253) -> (w246:dbl[])
      n97 = Number To Fractional String(number=w238, precision (6)=i16 15) -> (F-format string=w233:string[])  [unwired: 2 in]
      n98 = Number To Fractional String(number=w246, precision (6)=i16 15) -> (F-format string=w232:string[])  [unwired: 2 in]
      n99 = Build Array (concatenate)(w232, w233) -> (w231:string[])
    }
    n100 = for {
      tunnel: w22 -> [w262]
      tunnel: "Results Base Path" -> [w258]
      tunnel: [w257] -> w24 mode=indexing
      tunnel: w20 -> [w256] mode=indexing
      i -> [w261]
      n101 = for {
        tunnel: w256 -> [w277] mode=indexing
        tunnel: [w268] -> w266 mode=concatenating
        workers-P: _ -> [_]
        i -> [w267]
        n102 = Unbundle By Name(w277) -> ("i"=w276:dbl[], "q"=w271:dbl[])
        n103 = Format Into String(format string="CH%d_i_", w267) -> (resulting string=w278:string)  [unwired: 2 in, 1 out]
        n104 = Number To Fractional String(number=w276, precision (6)=i16 15) -> (F-format string=w280:string[])  [unwired: 2 in]
        n105 = Format Into String(format string="CH%d_q_", w267) -> (resulting string=w275:string)  [unwired: 2 in, 1 out]
        n106 = Number To Fractional String(number=w271, precision (6)=i16 15) -> (F-format string=w273:string[])  [unwired: 2 in]
        n107 = Build Array (concatenate)(w278, w280) -> (w269:string[])
        n108 = Build Array (concatenate)(w275, w273) -> (w270:string[])
        n109 = Build Array(w269, w270) -> (w268:string[][])
      }
      n110 = Format Into String(format string="_Run%d.csv", initial string=w262, w261) -> (resulting string=w260:string)  [unwired: 1 in, 1 out]
      n111 = Build Path(base path=w258, name or relative path=w260) -> (appended path=w259:path)
      n112 = call-poly <vilib>:"Write Delimited Spreadsheet.vi"("file path (dialog if empty)"=w259, "2D data"=w266, "transpose? (no:F)"=TRUE, "delimiter (\\t)"="," ("delimiter (\\t)")) -> ("error out"=w257:errorcluster)  [unwired: 10 in, 1 out]
    }
    n113 = Merge Errors(w24) -> (→"error out 3":errorcluster)
    n114 = Concatenate Strings(w22, "_Results.csv" ("string")) -> (w27:string)
    n115 = Build Path(base path="Results Base Path", name or relative path=w27) -> (appended path=w26:path)
    n116 = Insert Into Array(array=w18, index (row)=0, new element=string[] ["TxRxChannel", "DDCDUCFrequency", "AmpStabilityMean", "AmpStabilityStdDev", "AmpStabilityPkPk", "PhaseStabilityMean", "PhaseStabilityStdDev", "PhaseStabilityPkPk"]) -> (w29:string[][])  [unwired: 1 in]
    n117 = call-poly <vilib>:"Write Delimited Spreadsheet.vi"("file path (dialog if empty)"=w26, "2D data"=w29, "transpose? (no:F)"=FALSE, "delimiter (\\t)"="," ("delimiter (\\t)")) -> ("error out"=→"error out 4":errorcluster)  [unwired: 10 in, 1 out]
    "Current Frequency Under Test" <- w19
  }
  "Results" <- w3
